vi "RF Characterization UI Merged.vi"() -> ()   [LabVIEW 2010]
uses:
  RF Characterization States.ctl
  Drivers/Motion/Motion_Gantry Position.ctl
  <vilib>/Utility/NIReport.llb/NI_report.lvclass
  Report Generation States.ctl
  <vilib>/Analysis/1siggen.llb/Ramp Pattern by Delta.vi
  <vilib>/Utility/NIReport.llb/Append Text Table to Report (wrap).vi
  <vilib>/Utility/NIReport.llb/Append Numeric Table to Report (wrap).vi
  <vilib>/Analysis/NI_AALBase.lvlib
panel:
  in  "Close":bool
  in  "stop":bool
  in  "Prev":bool
  in  "Next":bool
  out "Main Tab Control":T1(tab)
  out "Gantry Moving Message":string="Gantry Moving"
  in  "Z":dbl min=-5.5 max=5.5 step=0.001 format="%.3g"
  in  "Y":dbl min=-5.5 max=5.5 step=0.001 format="%.3g"
  in  "X":dbl min=0.0 max=22.0 step=0.001 format="%.3g"
  in  "Gantry TCP address:port":string="192.168.0.3:502"
  in  "MICS ID":u32 format="%06.0x"
  in  "MICS Dongle Port":refnum<visa-resource-name>="COM5"
  in  "Start Attenuation Test":bool
  in  "Attenuation Samples":i32(knob)=1 caption="Samples" min=1 max=30 step=1 scale=1.0..30.0
  in  "Attenuation Increment":dbl(knob)=0.25 caption="Increment" min=0.25 max=5.0 step=0.25 scale=0.25..5.0
  in  "Attenuation Range":cluster{dbl, dbl}(slide)={0.0, 1.4141414141414141} caption="Range" scale=0.0..30.0
  out "Attenuation Graph":cluster{dbl, dbl}[](graph)
  out "Attenuation Cutoff (dB)":dbl=12.5
  out "MICS Power Graph":cluster{dbl, dbl}[](graph)
  in  "Power Range":cluster{dbl, dbl}(slide) caption="Range" scale=0.0..64.0
  in  "Power Increment":dbl(knob)=1.0 caption="Increment" min=1.0 max=5.0 step=1.0 scale=1.0..5.0
  in  "Power Samples":i32(knob)=1 caption="Samples" min=1 max=30 step=1 scale=1.0..30.0
  in  "Start Power Test":bool
  out "Power Cutoff":i32=12 format="%.0x"
  in  "Z-Layer":dbl(slide) min=0.0 max=0.0 step=1.0 scale=-5.5..5.5
  in  "X Range":cluster{"Min":dbl, "Max":dbl, "Increment":dbl}={"Min"=1.0, "Max"=20.0, "Increment"=0.25}
  in  "Y Range":cluster{"Min":dbl, "Max":dbl, "Increment":dbl}={"Min"=-5.0, "Max"=5.0, "Increment"=0.25}
  in  "Z Range":cluster{"Min":dbl, "Max":dbl, "Increment":dbl}={"Min"=0.0, "Max"=0.0, "Increment"=1.0}
  out "RF Mapping Graph":dbl[][](graph)
  in  "Mapping Samples":i32(knob)=1 caption="Samples" min=1 max=30 step=1 scale=1.0..30.0
  in  "Start RF Mapping":bool
  in  "WebBrowser":refnum<k7>(container)
  in  "Save Report":bool
  # "Gantry Configuration"
  # "MICS Configuration"
  # "Instructions:"
  # "Instructions:"
  # "Instructions:\nLorem ipsum veritas quo\nLorem ipsum veritas quo\nLorem ipsum veritas quo\nLorem ipsum veritas quo\nLorem ipsum veritas quo\nLorem ipsum veritas quo\nLorem ipsum veritas quo\nLorem ipsum veritas quo\nLorem ipsum veritas quo"
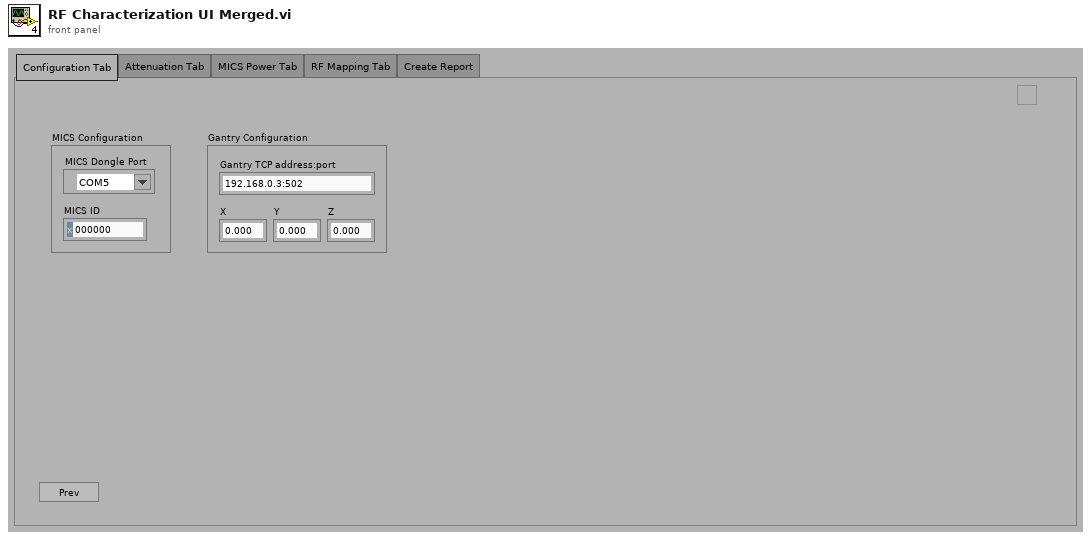
[diagram p1: front panel]
types:
  T1 = enum32{"Configuration Tab", "Attenuation Tab", "MICS Power Tab", "RF Mapping Tab", "Create Report"}
  T2 = typedef "RF Characterization States.ctl" = enum16{"Initialize", "Enable/Disable Navigation", "Set Next Action", "Set Prev Action", "Set Stop Action", "Prev Action Triggered", "Next Action Triggered", "Stop Action Triggered", "Move Gantry to Position", "Display Configuration Tab", "Check Configuration", "Display Attenuation Tab", "Check Attenuation Config", "Start Attenuation Test", "Check Attenuation Results", "Display Power Tab", "Check Power Config", "Start Power Test", "Check Power Results", "Display Mapping Tab", "Check Mapping Config", "Start Mapping Test", "Take Mapping Sample", "Finish Mapping Test", "Check Mapping Results", "Display Report Tab", "Generate Report", "Save Report", "Error", "Shutdown"}
  T3 = typedef "Motion_Gantry Position.ctl" = cluster{"Gantry Accel/Decel":dbl, "Gantry Velocity":dbl, "X-Position":dbl, "Y-Position":dbl, "Z-Position":dbl}
  T4 = cluster{"Next Action":cluster{"Action":T2, "Payload":variant}, "Prev Action":cluster{"Action":T2, "Payload":variant}, "Stop Action":cluster{"Action":T2, "Payload":variant}, "Configuration":cluster{"MICS Dongle Port":refnum<visa-resource-name>, "MICS ID":u32, "Gantry TCP address:port":string, "X-Position":dbl, "Y-Position":dbl, "Z-Position":dbl}, "Attenuation Config":cluster{"Range":cluster{dbl, dbl}, "Increment":dbl, "Samples":i32}, "Attenuation Results":cluster{dbl, dbl}[], "Attenuation Cutoff (dB)":dbl, "Power Config":cluster{"Range":cluster{dbl, dbl}, "Increment":dbl, "Samples":i32}, "Power Results":cluster{dbl, dbl}[], "Power Cutoff":u8, "Mapping Config":cluster{"Samples":i32, "X Range":cluster{"Min":dbl, "Max":dbl, "Increment":dbl}, "Y Range":cluster{"Min":dbl, "Max":dbl, "Increment":dbl}, "Z Range":cluster{"Min":dbl, "Max":dbl, "Increment":dbl}, "Positions":T3[], "Indices":cluster{i32, i32, i32}[]}, "Mapping Results":dbl[][][], "Refnums":cluster{"MICS Refnum":refnum<visa-resource-name>, "Motion Refnum":refnum<k5>}, "Mapping Index":i32, "Temp Report Path":path, "Previous Start Path":path, "Report":refnum<class "NI_report.lvclass">}
  T5 = enum8{"Enabled", "Disabled", "Disabled and Grayed Out"}
  T6 = cluster{"Prev Button":cluster{"Visible":bool, "Enable":enum8{"Enabled", "Disabled", "Disabled and Grayed Out"}}, "Next Button":cluster{"Visible":bool, "Enable":enum8{"Enabled", "Disabled", "Disabled and Grayed Out"}}, "Stop Button":cluster{"Visible":bool, "Enable":enum8{"Enabled", "Disabled", "Disabled and Grayed Out"}}}
  T7 = enum32{"Configuration Tab", "Attenuation Tab", "MICS Power Tab", "RF Mapping Tab"}
  T8 = typedef "Report Generation States.ctl" = enum16{"Initialize", "Generate Header", "Generate Summary", "Generate Attenuation Section", "Generate MICS Power Section", "Generate RF Mapping Section 1", "Generate RF Mapping Section 2", "Show Report in UI"}
  T9 = enum16{"Standard Report", "HTML", "Word", "Excel"}
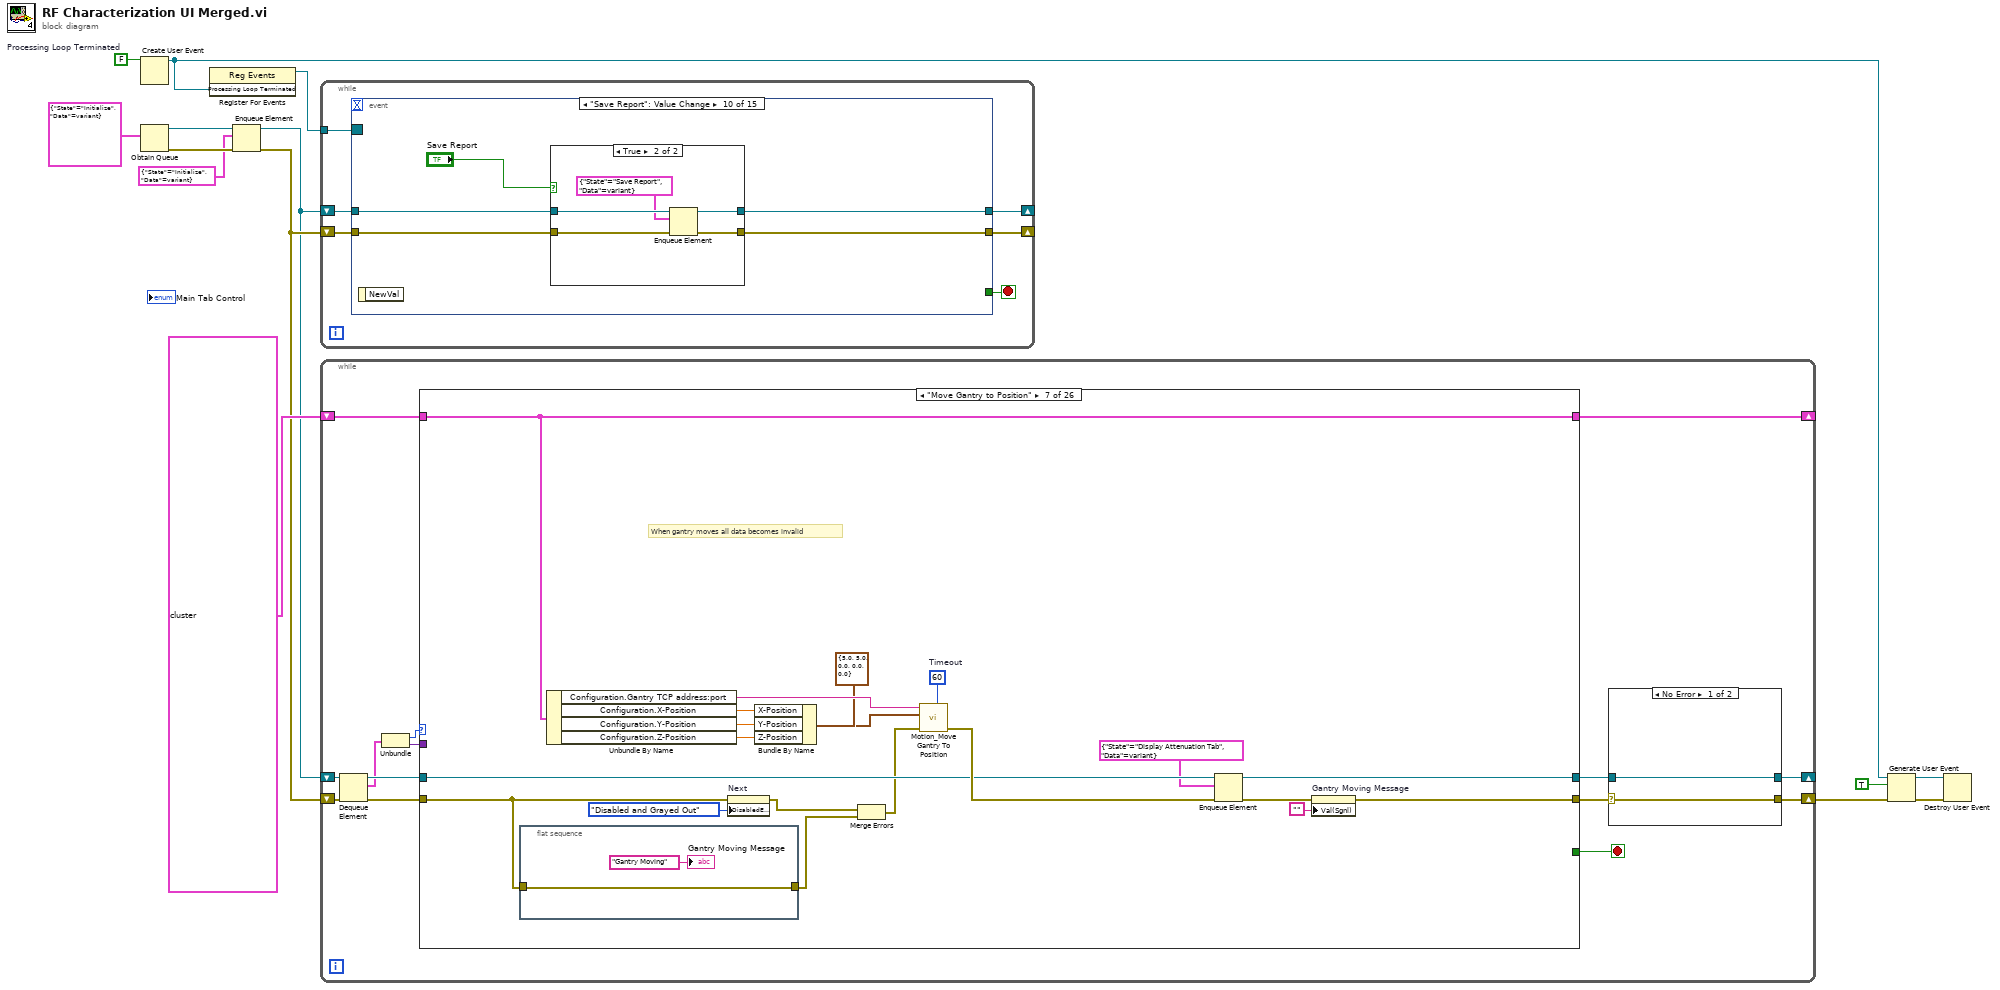
[diagram p0: block diagram]
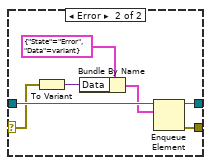
[diagram p2: hidden frame]
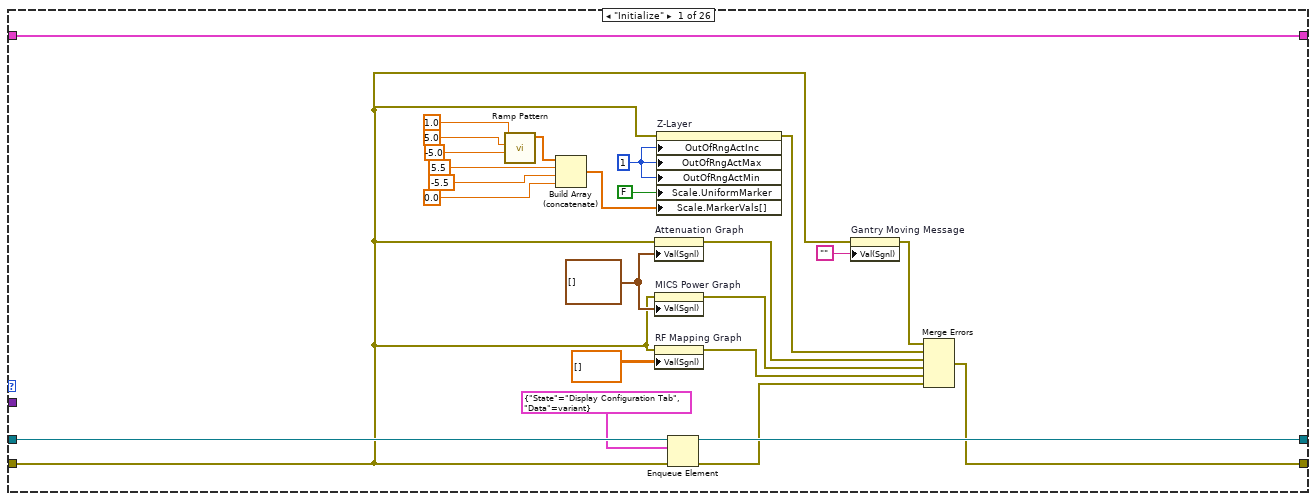
[diagram p3: hidden frame]
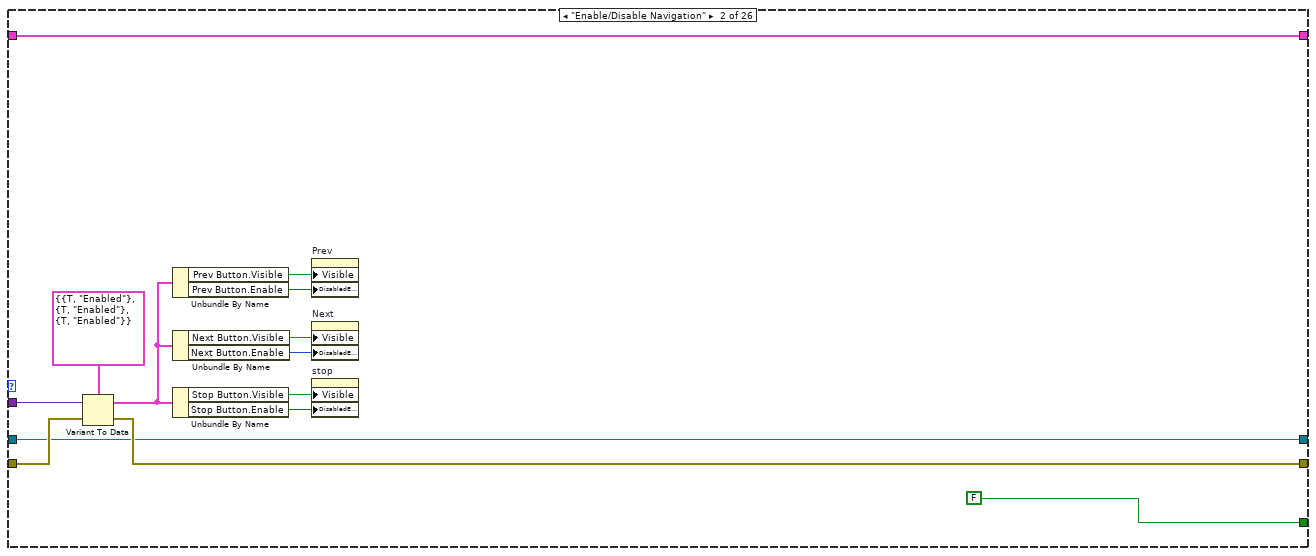
[diagram p4: hidden frame]
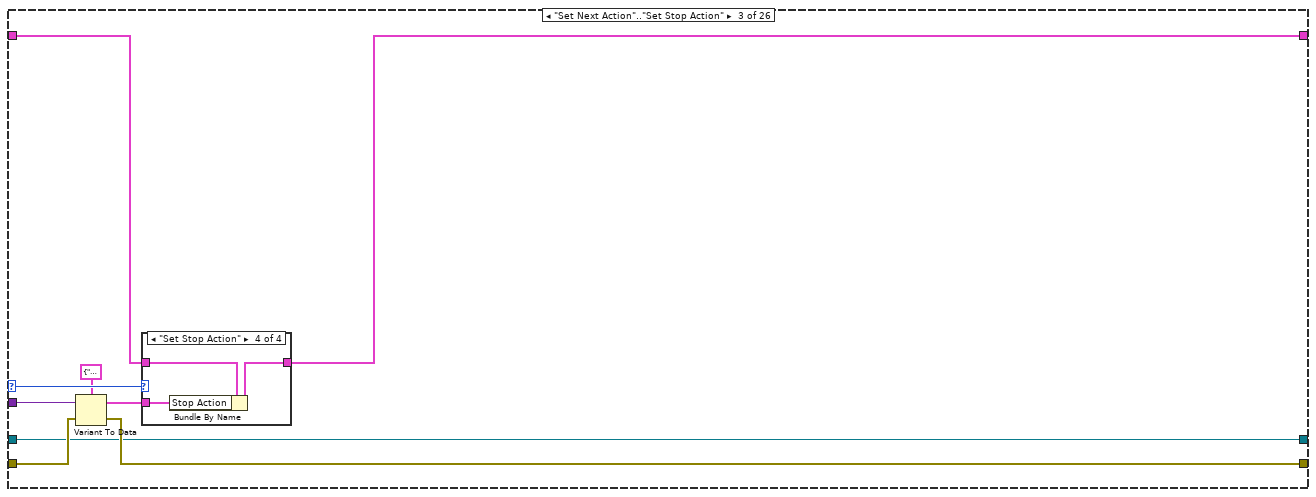
[diagram p5: hidden frame]
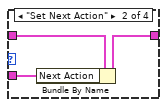
[diagram p7: hidden frame]
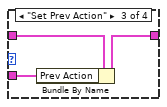
[diagram p8: hidden frame]
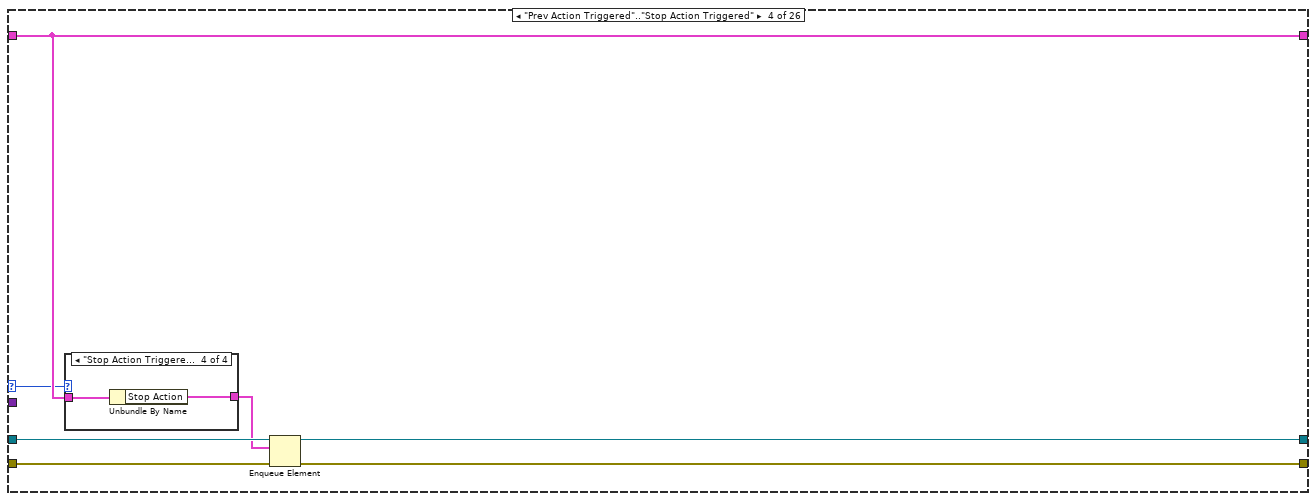
[diagram p9: hidden frame]
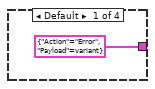
[diagram p10: hidden frame]
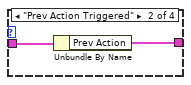
[diagram p11: hidden frame]
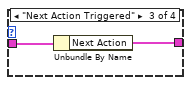
[diagram p12: hidden frame]
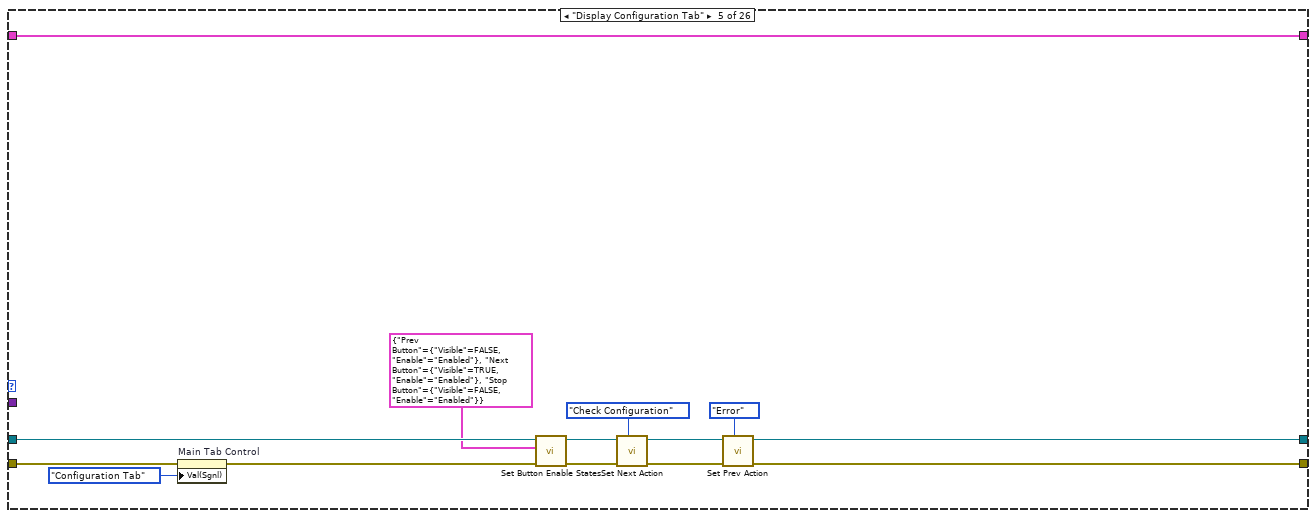
[diagram p13: hidden frame]
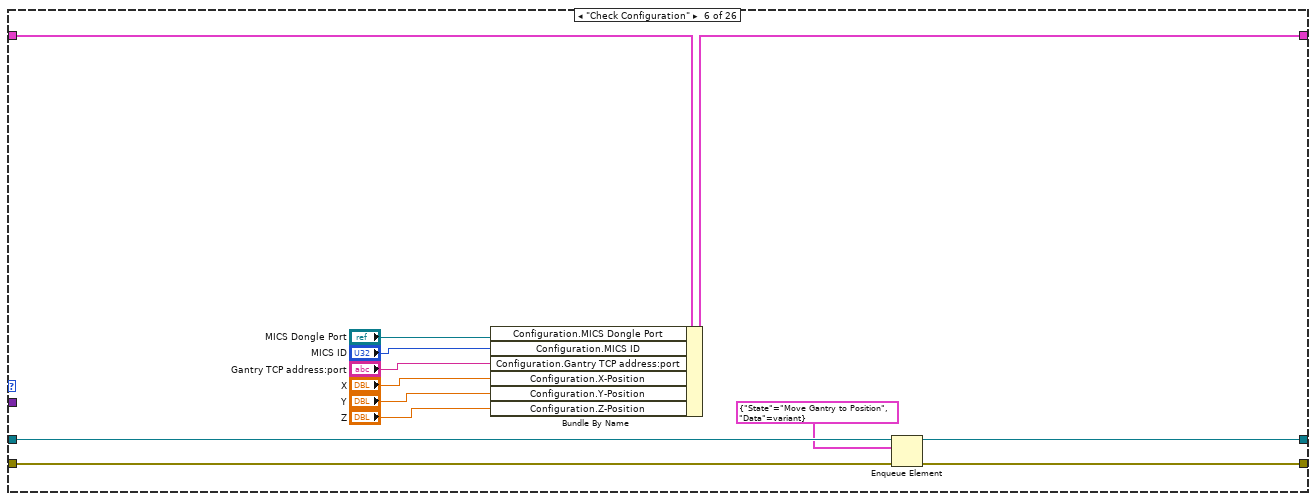
[diagram p14: hidden frame]
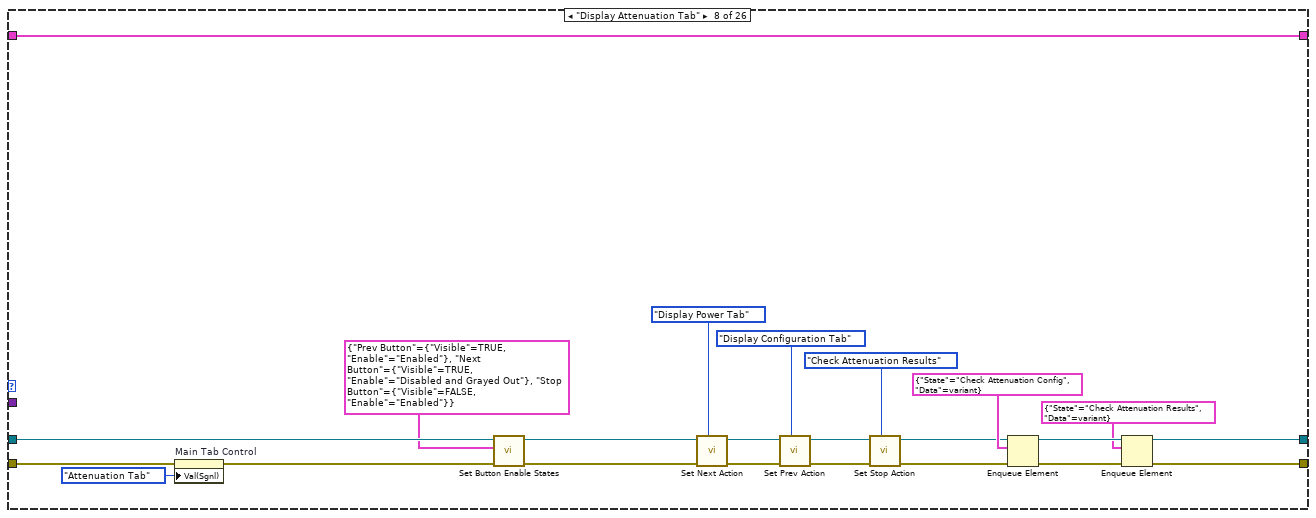
[diagram p15: hidden frame]
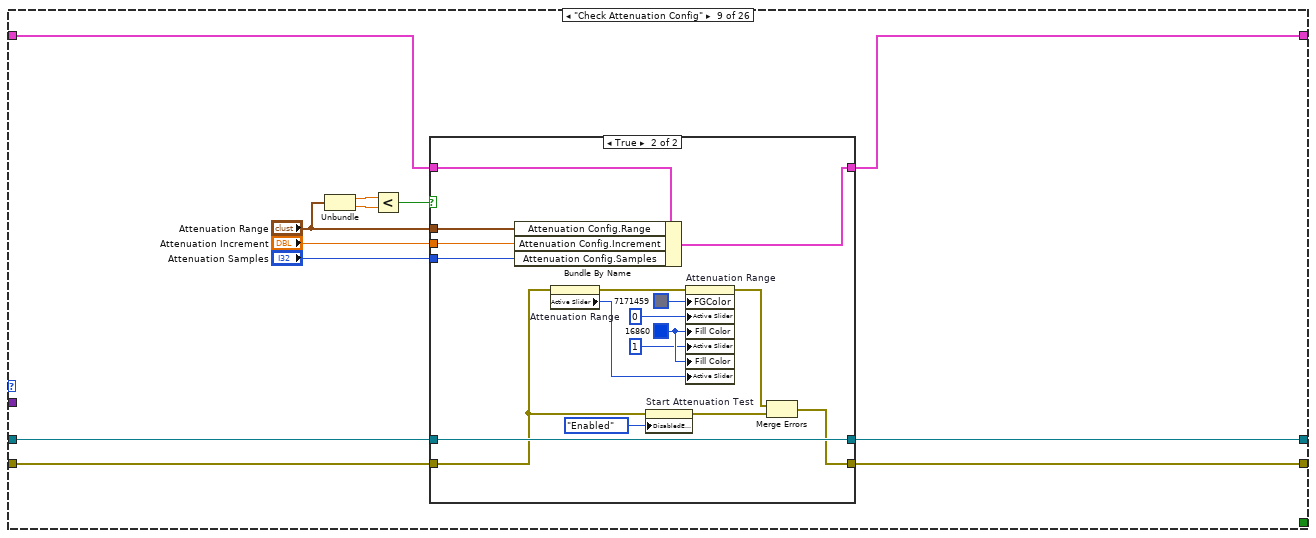
[diagram p16: hidden frame]
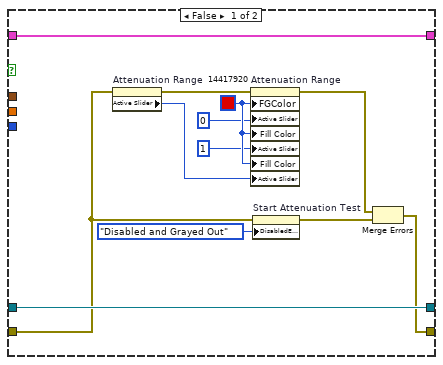
[diagram p17: hidden frame]
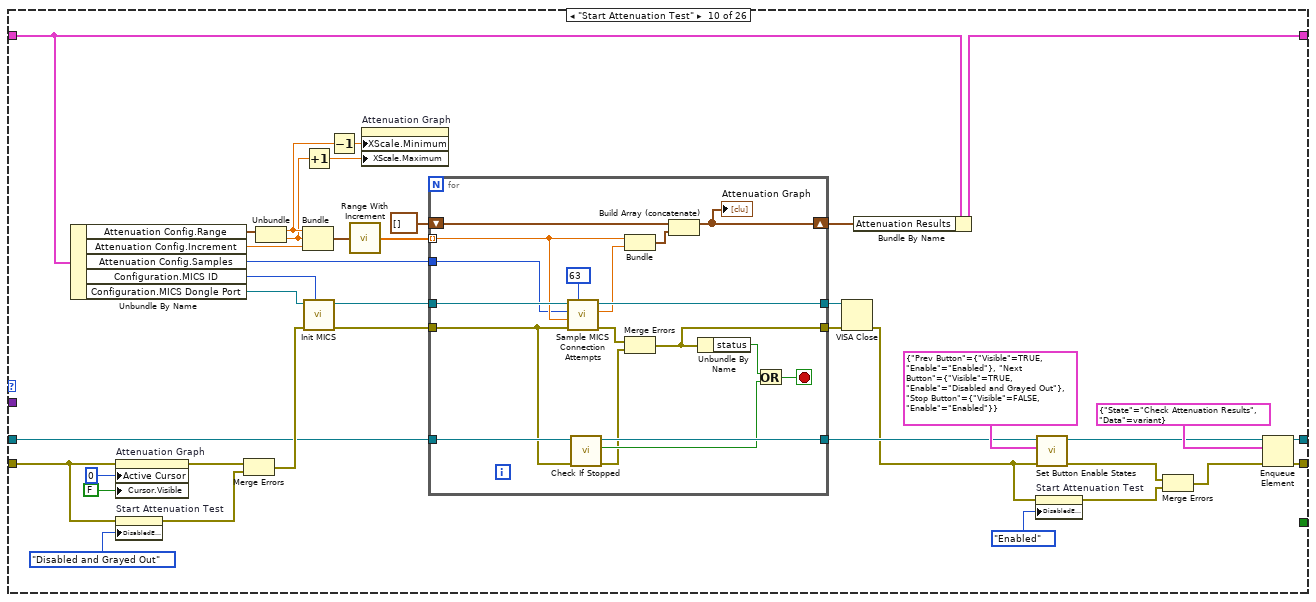
[diagram p18: hidden frame]
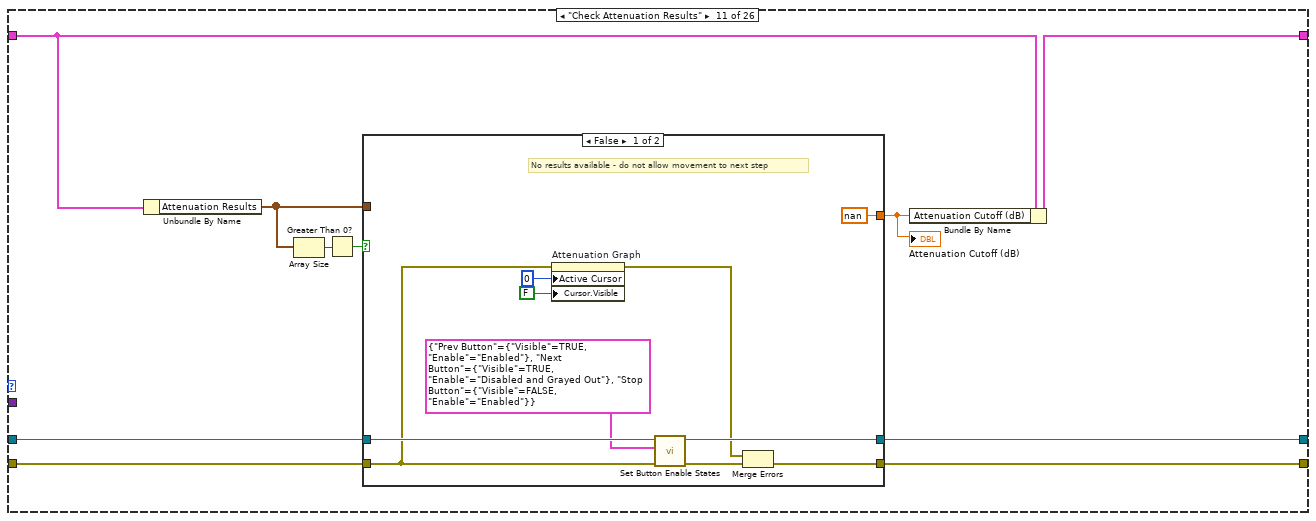
[diagram p19: hidden frame]
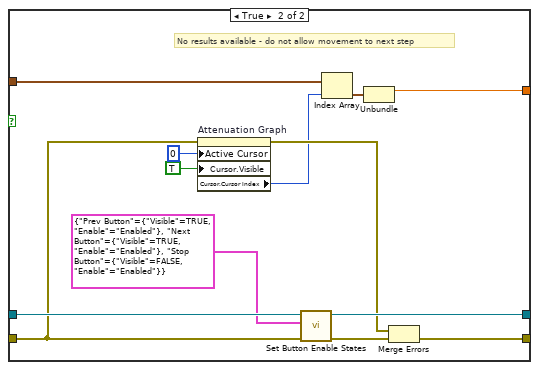
[diagram p20: hidden frame]
diagram:
  w11 = FALSE  # Processing Loop Terminated
  n1 = Create User Event(user event datatype=w11) -> (user event=w8:refnum<user-event>)  [unwired: 1 in, 1 out]
  n2 = Obtain Queue(element data type=cluster{"State":T2, "Data":variant} {"State"=enum."Initialize", "Data"=variant}) -> (queue out=w3:refnum<queue>, error out=w12:errorcluster)  [unwired: 4 in, 1 out]
  n3 = register-events(w8) -> (reference out=w10:refnum<event-registration>)  [unwired: 2 in, 1 out]
  n4 = Enqueue Element(queue=w3, element=cluster{"State":T2, "Data":variant} {"State"=enum."Initialize", "Data"=variant}, error in (no error)=w12) -> (queue out=w2:refnum<queue>, error out=w4:errorcluster)  [unwired: 1 in, 1 out]
  n5 = while {
    shift-right: [w19] -> _
    shift-left: w2 -> [w20]
    shift-right: [w17] -> _
    shift-left: w4 -> [w18]
    tunnel: w10 -> [w16]
    stop <- w15 stop-if-true
    n6 = event shown="[9] \"Save Report\": Value Change" {
      selector: w16 -> [_ _ _ _ _ _ _ _ _ _ _ _ _ _ _]
      dyn-events: _ -> [_ _ _ _ _ _ _ _ _ _ _ _ _ _ _]
      timeout: _ -> [_ _ _ _ _ _ _ _ _ _ _ _ _ _ _]
      tunnel: w20 -> [w22 w24 w30 w43 w55 w67 w80 w96 w107 w120 w132 w137 w141 w145 w150]
      tunnel: [w22 w24 w28 w41 w54 w65 w77 w93 w105 w118 w129 w134 w139 w144 w149] -> w19
      tunnel: w18 -> [w21 w23 w29 w40 w53 w66 w78 w94 w106 w119 w130 w135 w140 w147 w152]
      tunnel: [w21 w23 w27 w39 w52 w64 w79 w95 w104 w117 w131 w136 w138 w146 w151] -> w17
      tunnel: [_ w25 TRUE ("Processing Loop Terminated") _ _ _ _ _ _ _ _ _ _ _ _] -> w15
      event Timeout {
        n7 = event-data() -> ()  [unwired: 1 in, 2 out]
      }
      event User Event {
        n8 = event-data() -> ("Processing Loop Terminated"=w25:bool)  [unwired: 1 in, 3 out]
      }
      event "Close": Value Change {
        n9 = event-data() -> ()  [unwired: 1 in, 1 out]
        n10 = case shown="True" "Close" {
          tunnel: w30 -> [w33 w37]
          tunnel: w29 -> [w32 w38]
          tunnel: [w33 w36] -> w28
          tunnel: [w32 w35] -> w27
          frame False {
          }
          frame True {
            n11 = Enqueue Element(queue=w37, element=cluster{"State":T2, "Data":variant} {"State"=enum."Shutdown", "Data"=variant}, error in (no error)=w38) -> (queue out=w36:refnum<queue>, error out=w35:errorcluster)  [unwired: 1 in, 1 out]
          }
        }
      }
      event "Next": Value Change {
        n12 = event-data() -> ()  [unwired: 1 in, 1 out]
        n13 = case shown="True" "Next" {
          tunnel: w43 -> [w45 w50]
          tunnel: [w45 w49] -> w41
          tunnel: w40 -> [w44 w48]
          tunnel: [w44 w47] -> w39
          frame False {
          }
          frame True {
            n14 = Enqueue Element(queue=w50, element=cluster{"State":T2, "Data":variant} {"State"=enum."Next Action Triggered", "Data"=variant}, error in (no error)=w48) -> (queue out=w49:refnum<queue>, error out=w47:errorcluster)  [unwired: 1 in, 1 out]
          }
        }
      }
      event "Prev": Value Change {
        n15 = event-data() -> ()  [unwired: 1 in, 1 out]
        n16 = case shown="True" "Prev" {
          tunnel: w55 -> [w57 w62]
          tunnel: [w57 w61] -> w54
          tunnel: w53 -> [w56 w60]
          tunnel: [w56 w59] -> w52
          frame False {
          }
          frame True {
            n17 = Enqueue Element(queue=w62, element=cluster{"State":T2, "Data":variant} {"State"=enum."Prev Action Triggered", "Data"=variant}, error in (no error)=w60) -> (queue out=w61:refnum<queue>, error out=w59:errorcluster)  [unwired: 1 in, 1 out]
          }
        }
      }
      event "stop": Value Change {
        n18 = event-data() -> ()  [unwired: 1 in, 1 out]
        n19 = case shown="True" "stop" {
          tunnel: w67 -> [w69 w76]
          tunnel: [w69 w75] -> w65
          tunnel: w66 -> [w68 w74]
          tunnel: [w68 w71] -> w64
          frame False {
          }
          frame True {
            n20 = Enqueue Element(queue=w76, element=cluster{"State":T2, "Data":variant} {"State"=enum."Stop Action Triggered", "Data"=variant}, error in (no error)=w74) -> (queue out=w75:refnum<queue>, error out=w72:errorcluster)  [unwired: 1 in, 1 out]
            n21 = property on="stop" class="Bool"(error in=w72, "DisabledEnum"=T5."Disabled and Grayed Out" ("Disabled")) -> (error out=w71:errorcluster)  [unwired: 1 in, 1 out]
          }
        }
      }
      event "Start Attenuation Test": Value Change {
        n22 = event-data() -> ()  [unwired: 1 in, 1 out]
        n23 = case shown="True" "Start Attenuation Test" {
          tunnel: w80 -> [w83 w88]
          tunnel: [w82 w91] -> w79
          tunnel: w78 -> [w82 w87]
          tunnel: [w83 w90] -> w77
          frame False {
          }
          frame True {
            n24 = call "Set Button Enable States.vi"("error in (no error)"=w87, "Button States"=T6 {"Prev Button"={"Visible"=TRUE, "Enable"=enum."Disabled and Grayed Out"}, "Next Button"={"Visible"=TRUE, "Enable"=enum."Disabled and Grayed Out"}, "Stop Button"={"Visible"=TRUE, "Enable"=enum."Enabled"}}, "queue in"=w88) -> ("error out"=w85:errorcluster, "queue out"=w86:refnum<queue>)  [unwired: 7 in]
            n25 = Enqueue Element(queue=w86, element=cluster{"State":T2, "Data":variant} {"State"=enum."Start Attenuation Test", "Data"=variant}, error in (no error)=w85) -> (queue out=w90:refnum<queue>, error out=w91:errorcluster)  [unwired: 1 in, 1 out]
          }
        }
      }
      event "Start Power Test": Value Change {
        n26 = event-data() -> ()  [unwired: 1 in, 1 out]
        n27 = case shown="True" "Start Power Test" {
          tunnel: w96 -> [w98 w101]
          tunnel: [w97 w102] -> w95
          tunnel: w94 -> [w97 w103]
          tunnel: [w98 w100] -> w93
          frame False {
          }
          frame True {
            n28 = Enqueue Element(queue=w101, element=cluster{"State":T2, "Data":variant} {"State"=enum."Start Power Test", "Data"=variant}, error in (no error)=w103) -> (queue out=w100:refnum<queue>, error out=w102:errorcluster)  [unwired: 1 in, 1 out]
          }
        }
      }
      event "Start RF Mapping": Value Change {
        n29 = event-data() -> ()  [unwired: 1 in, 1 out]
        n30 = case shown="True" "Start RF Mapping" {
          tunnel: w107 -> [w110 w115]
          tunnel: w106 -> [w109 w114]
          tunnel: [w110 w112] -> w105
          tunnel: [w109 w111] -> w104
          frame False {
          }
          frame True {
            n31 = Enqueue Element(queue=w115, element=cluster{"State":T2, "Data":variant} {"State"=enum."Start Mapping Test", "Data"=variant}, error in (no error)=w114) -> (queue out=w112:refnum<queue>, error out=w111:errorcluster)  [unwired: 1 in, 1 out]
          }
        }
      }
      event "Save Report": Value Change {
        n32 = event-data() -> ()  [unwired: 1 in, 1 out]
        n33 = case shown="True" "Save Report" {
          tunnel: w120 -> [w122 w127]
          tunnel: w119 -> [w121 w126]
          tunnel: [w122 w124] -> w118
          tunnel: [w121 w123] -> w117
          frame False {
          }
          frame True {
            n34 = Enqueue Element(queue=w127, element=cluster{"State":T2, "Data":variant} {"State"=enum."Save Report", "Data"=variant}, error in (no error)=w126) -> (queue out=w124:refnum<queue>, error out=w123:errorcluster)  [unwired: 1 in, 1 out]
          }
        }
      }
      event "Attenuation Range", "Attenuation Increment", "Attenuation Samples": Value Change {
        n35 = event-data() -> ()  [unwired: 1 in, 1 out]
        n36 = Enqueue Element(queue=w132, element=cluster{"State":T2, "Data":variant} {"State"=enum."Check Attenuation Config", "Data"=variant}, error in (no error)=w130) -> (queue out=w129:refnum<queue>, error out=w131:errorcluster)  [unwired: 1 in, 1 out]
      }
      event "Attenuation Graph": Cursor Move {
        n37 = event-data() -> ()  [unwired: 1 in, 1 out]
        n38 = Enqueue Element(queue=w137, element=cluster{"State":T2, "Data":variant} {"State"=enum."Check Attenuation Results", "Data"=variant}, error in (no error)=w135) -> (queue out=w134:refnum<queue>, error out=w136:errorcluster)  [unwired: 1 in, 1 out]
      }
      event "Power Range", "Power Increment", "Power Samples": Value Change {
        n39 = event-data() -> ()  [unwired: 1 in, 1 out]
        n40 = Enqueue Element(queue=w141, element=cluster{"State":T2, "Data":variant} {"State"=enum."Check Power Config", "Data"=variant}, error in (no error)=w140) -> (queue out=w139:refnum<queue>, error out=w138:errorcluster)  [unwired: 1 in, 1 out]
      }
      event "MICS Power Graph": Cursor Move {
        n41 = event-data() -> ()  [unwired: 1 in, 1 out]
        n42 = Enqueue Element(queue=w145, element=cluster{"State":T2, "Data":variant} {"State"=enum."Check Power Results", "Data"=variant}, error in (no error)=w147) -> (queue out=w144:refnum<queue>, error out=w146:errorcluster)  [unwired: 1 in, 1 out]
      }
      event "Z-Layer": Value Change {
        n43 = event-data() -> ()  [unwired: 1 in, 1 out]
        n44 = Enqueue Element(queue=w150, element=cluster{"State":T2, "Data":variant} {"State"=enum."Check Mapping Results", "Data"=variant}, error in (no error)=w152) -> (queue out=w149:refnum<queue>, error out=w151:errorcluster)  [unwired: 1 in, 1 out]
      }
    }
  }
  n45 = while {
    shift-right: [w154] -> w9
    shift-left: w4 -> [w165]
    shift-right: [w153] -> _
    shift-left: w2 -> [w166]
    shift-right: [w159] -> _
    shift-left: T4 {"Next Action"={"Action"=enum."Error", "Payload"=variant}, "Prev Action"={"Action"=enum."Error", "Payload"=variant}, "Stop Action"={"Action"=enum."Error", "Payload"=variant}, "Configuration"={"MICS Dongle Port"="", "MICS ID"=0, "Gantry TCP address:port"="", "X-Position"=0.0, "Y-Position"=0.0, "Z-Position"=0.0}, "Attenuation Config"={"Range"={0.0, 0.0}, "Increment"=0.0, "Samples"=0}, "Attenuation Results"=[], "Attenuation Cutoff (dB)"=0.0, "Power Config"={"Range"={0.0, 0.0}, "Increment"=0.0, "Samples"=0}, "Power Results"=[], "Power Cutoff"=0, "Mapping Config"={"Samples"=0, "X Range"={"Min"=0.0, "Max"=0.0, "Increment"=0.0}, "Y Range"={"Min"=0.0, "Max"=0.0, "Increment"=0.0}, "Z Range"={"Min"=0.0, "Max"=0.0, "Increment"=0.0}, "Positions"=[], "Indices"=[]}, "Mapping Results"=[], "Refnums"={"MICS Refnum"="", "Motion Refnum"=refnum}, "Mapping Index"=0, "Temp Report Path"=path "", "Previous Start Path"=path "", "Report"=refnum} -> [w160]
    stop <- w157 stop-if-true
    n46 = Dequeue Element(queue=w166, error in (no error)=w165) -> (queue out=w164:refnum<queue>, element=w163:cluster{"State":T2, "Data":variant}, error out=w158:errorcluster)  [unwired: 1 in, 1 out]
    n47 = Unbundle(w163) -> ("State"=w162:T2, "Data"=w161:variant)
    n48 = case shown="\"Move Gantry to Position\"" w162 {
      selector: w162 -> [_ _ w218 w234 _ _ _ _ _ _ _ _ _ _ _ _ _ _ _ _ _ _ _ _ _ _]
      tunnel: [w191 w207 w221 w235 w255 w265 w276 w305 w320 w383 w421 w450 w478 w538 w576 w606 w629 w643 w694 w726 w751 w756 w777 w1010 w1044 w1054] -> w156
      tunnel: w164 -> [w199 w206 w217 w240 w252 w264 w291 w315 w323 w362 w424 w452 w481 w517 w579 w609 w630 w642 w687 w732 w752 w760 w779 w1009 w1043 w1055]
      tunnel: w161 -> [_ w213 w223 _ _ _ _ _ _ _ _ _ _ _ _ _ _ _ _ _ _ _ _ _ w1041 _]
      tunnel: [_ FALSE _ _ _ _ _ _ _ _ _ _ _ _ _ _ _ _ _ _ _ _ _ _ _ TRUE] -> w157
      tunnel: [w198 w206 w217 w236 w257 w263 w290 w303 w321 w382 w422 w451 w479 w537 w577 w607 w630 w644 w693 w727 w752 w754 w779 w1009 w1042 w1055] -> w155
      tunnel: w160 -> [w200 w205 w220 w238 w261 w268 w294 w319 w329 w385 w419 w472 w474 w540 w574 w628 w631 w654 w709 w737 w749 w757 w774 w1020 w1045 w1056]
      tunnel: [w200 w205 w219 w238 w261 w267 w294 w319 w328 w384 w418 w472 w473 w539 w573 w628 w631 w636 w708 w737 w749 w757 w778 w1020 w1045 w1056] -> w159
      tunnel: w158 -> [w178 w208 w222 w239 w259 w266 w281 w318 w322 w361 w423 w453 w480 w516 w578 w608 w629 w650 w715 w735 w751 w770 w776 w1018 w1039 w1054]
      frame "Initialize" {
        w190 = u8 1 ("Response to Value Outside Limits:Increment")
        w196 = cluster{dbl, dbl}[] [] ("Value (Signaling)")
        n49 = call-poly <vilib>:"Ramp Pattern.vi"("start"=-5.0, "end"=5.0, "delta"=1.0) -> ("Ramp Pattern"=w188:dbl[])  [unwired: 6 in, 2 out]
        n50 = Build Array (concatenate)(w188, 5.5 ("delta"), -5.5 ("delta"), 0.0 ("delta")) -> (w181:dbl[])
        n51 = property on="Attenuation Graph" class="XYGraph (strict)"(error in=w178, "Val(Sgnl)"=w196) -> (error out=w177:errorcluster)  [unwired: 1 in, 1 out]
        n52 = property on="MICS Power Graph" class="XYGraph (strict)"(error in=w178, "Val(Sgnl)"=w196) -> (error out=w193:errorcluster)  [unwired: 1 in, 1 out]
        n53 = property on="RF Mapping Graph" class="IntGraph (strict)"(error in=w178, "Val(Sgnl)"=dbl[][] [] ("Value (Signaling)")) -> (error out=w194:errorcluster)  [unwired: 1 in, 1 out]
        n54 = property on="Z-Layer" class="Slide (strict)"(error in=w178, "OutOfRngActInc"=w190, "OutOfRngActMax"=w190, "OutOfRngActMin"=w190, "Scale.UniformMarker"=FALSE ("Scale.Uniform Marker Spacing?"), "Scale.MarkerVals[]"=w181) -> (error out=w180:errorcluster)  [unwired: 1 in, 1 out]
        n55 = Enqueue Element(queue=w199, element=cluster{"State":T2, "Data":variant} {"State"=enum."Display Configuration Tab", "Data"=variant}, error in (no error)=w178) -> (queue out=w198:refnum<queue>, error out=w192:errorcluster)  [unwired: 1 in, 1 out]
        n56 = property on="Gantry Moving Message" class="Str"(error in=w178, "Val(Sgnl)"="") -> (error out=w179:errorcluster)  [unwired: 1 in, 1 out]
        n57 = Merge Errors(w179, w180, w177, w193, w194, w192) -> (w191:errorcluster)
      }
      frame "Enable/Disable Navigation" {
        n58 = Variant To Data(error in=w208, Variant=w213, type=T6 {"Prev Button"={"Visible"=TRUE, "Enable"=enum."Enabled"}, "Next Button"={"Visible"=TRUE, "Enable"=enum."Enabled"}, "Stop Button"={"Visible"=TRUE, "Enable"=enum."Enabled"}} ("Button States")) -> (error out=w207:errorcluster, data=w203:T6)
        n59 = Unbundle By Name(w203) -> ("Prev Button.Visible"=w212:bool, "Prev Button.Enable"=w211:T5)
        n60 = Unbundle By Name(w203) -> ("Next Button.Visible"=w210:bool, "Next Button.Enable"=w209:T5)
        n61 = Unbundle By Name(w203) -> ("Stop Button.Visible"=w202:bool, "Stop Button.Enable"=w201:T5)
        n62 = property on="Prev" class="Bool"("Visible"=w212, "DisabledEnum"=w211) -> ()  [unwired: 2 in, 2 out]
        n63 = property on="Next" class="Bool"("Visible"=w210, "DisabledEnum"=w209) -> ()  [unwired: 2 in, 2 out]
        n64 = property on="stop" class="Bool"("Visible"=w202, "DisabledEnum"=w201) -> ()  [unwired: 2 in, 2 out]
      }
      frame "Set Next Action".."Set Stop Action" {
        n65 = Variant To Data(error in=w222, Variant=w223, type=cluster{"Action":T2, "Payload":variant} {"Action"=enum."Error", "Payload"=variant} ("Action")) -> (error out=w221:errorcluster, data=w215:cluster{"Action":T2, "Payload":variant})
        n66 = case shown="\"Set Stop Action\"" w218 {
          tunnel: w215 -> [_ w227 w230 w233]
          tunnel: w220 -> [w224 w226 w229 w232]
          tunnel: [w224 w225 w228 w231] -> w219
          frame Default {
          }
          frame "Set Next Action" {
            n67 = Bundle By Name(cluster=w226, "Next Action"=w227) -> (w225:T4)
          }
          frame "Set Prev Action" {
            n68 = Bundle By Name(cluster=w229, "Prev Action"=w230) -> (w228:T4)
          }
          frame "Set Stop Action" {
            n69 = Bundle By Name(cluster=w232, "Stop Action"=w233) -> (w231:T4)
          }
        }
      }
      frame "Prev Action Triggered".."Stop Action Triggered" {
        n70 = case shown="\"Stop Action Triggered\"" w234 {
          tunnel: w238 -> [_ w243 w245 w247]
          tunnel: [cluster{"Action":T2, "Payload":variant} {"Action"=enum."Error", "Payload"=variant} ("Prev Action") w242 w244 w246] -> w237
          frame Default {
          }
          frame "Prev Action Triggered" {
            n71 = Unbundle By Name(w243) -> ("Prev Action"=w242:cluster{"Action":T2, "Payload":variant})
          }
          frame "Next Action Triggered" {
            n72 = Unbundle By Name(w245) -> ("Next Action"=w244:cluster{"Action":T2, "Payload":variant})
          }
          frame "Stop Action Triggered" {
            n73 = Unbundle By Name(w247) -> ("Stop Action"=w246:cluster{"Action":T2, "Payload":variant})
          }
        }
        n74 = Enqueue Element(queue=w240, element=w237, error in (no error)=w239) -> (queue out=w236:refnum<queue>, error out=w235:errorcluster)  [unwired: 1 in, 1 out]
      }
      frame "Display Configuration Tab" {
        n75 = property on="Main Tab Control" class="TabCtl (strict)"(error in=w259, "Val(Sgnl)"=T7."Configuration Tab" ("Value (Signaling)")) -> (error out=w251:errorcluster)  [unwired: 1 in, 1 out]
        n76 = call "Set Button Enable States.vi"("error in (no error)"=w251, "Button States"=T6 {"Prev Button"={"Visible"=FALSE, "Enable"=enum."Enabled"}, "Next Button"={"Visible"=TRUE, "Enable"=enum."Enabled"}, "Stop Button"={"Visible"=FALSE, "Enable"=enum."Enabled"}}, "queue in"=w252) -> ("error out"=w250:errorcluster, "queue out"=w249:refnum<queue>)  [unwired: 7 in]
        n77 = call "Set Next Action.vi"("Action"=RF_Characterization_States."Check Configuration", "error in (no error)"=w250, "queue in"=w249) -> ("error out"=w256:errorcluster, "queue out"=w258:refnum<queue>)  [unwired: 7 in]
        n78 = call "Set Prev Action.vi"("Action"=RF_Characterization_States."Error", "error in (no error)"=w256, "queue in"=w258) -> ("error out"=w255:errorcluster, "queue out"=w257:refnum<queue>)  [unwired: 7 in]
      }
      frame "Check Configuration" {
        n79 = Bundle By Name(cluster=w268, "Configuration.MICS Dongle Port"="MICS Dongle Port", "Configuration.MICS ID"="MICS ID", "Configuration.Gantry TCP address:port"="Gantry TCP address:port", "Configuration.X-Position"="X", "Configuration.Y-Position"="Y", "Configuration.Z-Position"="Z") -> (w267:T4)
        n80 = Enqueue Element(queue=w264, element=cluster{"State":T2, "Data":variant} {"State"=enum."Move Gantry to Position", "Data"=variant}, error in (no error)=w266) -> (queue out=w263:refnum<queue>, error out=w265:errorcluster)  [unwired: 1 in, 1 out]
      }
      frame "Move Gantry to Position" {
        w283 = 60  # Timeout
        # "When gantry moves all data becomes invalid"
        n81 = flat-sequence {
          tunnel: w281 -> [w296]
          tunnel: [w296] -> w280
          frame #0 {
            "Gantry Moving Message" <- "Gantry Moving" ("Gantry Moving Message")
          }
        }
        n82 = Unbundle By Name(w294) -> ("Configuration.Gantry TCP address:port"=w293:string, "Configuration.X-Position"=w287:dbl, "Configuration.Y-Position"=w286:dbl, "Configuration.Z-Position"=w285:dbl)
        n83 = property on="Next" class="Bool"(error in=w281, "DisabledEnum"=T5."Disabled and Grayed Out" ("Disabled")) -> (error out=w279:errorcluster)  [unwired: 1 in, 1 out]
        n84 = Bundle By Name(cluster=T3 {"Gantry Accel/Decel"=5.0, "Gantry Velocity"=5.0, "X-Position"=0.0, "Y-Position"=0.0, "Z-Position"=0.0} ("Gantry Move Data"), "X-Position"=w287, "Y-Position"=w286, "Z-Position"=w285) -> (w284:T3)
        n85 = Merge Errors(w279, w280) -> (w278:errorcluster)
        n86 = call "Motion_Move Gantry To Position.vi"("Timeout sec (-1 = No timeout)"=w283, "error in"=w278, "Gantry Move Data"=w284, "TCP address:port"=w293) -> ("error out"=w292:errorcluster)  [unwired: 6 in, 1 out]
        n87 = Enqueue Element(queue=w291, element=cluster{"State":T2, "Data":variant} {"State"=enum."Display Attenuation Tab", "Data"=variant}, error in (no error)=w292) -> (queue out=w290:refnum<queue>, error out=w277:errorcluster)  [unwired: 1 in, 1 out]
        n88 = property on="Gantry Moving Message" class="Str"(error in=w277, "Val(Sgnl)"="") -> (error out=w276:errorcluster)  [unwired: 1 in, 1 out]
      }
      frame "Display Attenuation Tab" {
        n89 = property on="Main Tab Control" class="TabCtl (strict)"(error in=w318, "Val(Sgnl)"=T1."Attenuation Tab" ("Value (Signaling)")) -> (error out=w314:errorcluster)  [unwired: 1 in, 1 out]
        n90 = call "Set Button Enable States.vi"("error in (no error)"=w314, "Button States"=T6 {"Prev Button"={"Visible"=TRUE, "Enable"=enum."Enabled"}, "Next Button"={"Visible"=TRUE, "Enable"=enum."Disabled and Grayed Out"}, "Stop Button"={"Visible"=FALSE, "Enable"=enum."Enabled"}}, "queue in"=w315) -> ("error out"=w317:errorcluster, "queue out"=w316:refnum<queue>)  [unwired: 7 in]
        n91 = call "Set Next Action.vi"("Action"=RF_Characterization_States."Display Power Tab", "error in (no error)"=w317, "queue in"=w316) -> ("error out"=w311:errorcluster, "queue out"=w312:refnum<queue>)  [unwired: 7 in]
        n92 = call "Set Prev Action.vi"("Action"=RF_Characterization_States."Display Configuration Tab", "error in (no error)"=w311, "queue in"=w312) -> ("error out"=w300:errorcluster, "queue out"=w301:refnum<queue>)  [unwired: 7 in]
        n93 = call "Set Stop Action.vi"("Action"=RF_Characterization_States."Check Attenuation Results", "error in (no error)"=w300, "queue in"=w301) -> ("error out"=w297:errorcluster, "queue out"=w298:refnum<queue>)  [unwired: 7 in]
        n94 = Enqueue Element(queue=w298, element=cluster{"State":T2, "Data":variant} {"State"=enum."Check Attenuation Config", "Data"=variant}, error in (no error)=w297) -> (queue out=w304:refnum<queue>, error out=w308:errorcluster)  [unwired: 1 in, 1 out]
        n95 = Enqueue Element(queue=w304, element=cluster{"State":T2, "Data":variant} {"State"=enum."Check Attenuation Results", "Data"=variant}, error in (no error)=w308) -> (queue out=w303:refnum<queue>, error out=w305:errorcluster)  [unwired: 1 in, 1 out]
      }
      frame "Check Attenuation Config" {
        n96 = Unbundle("Attenuation Range") -> (w326:dbl, w325:dbl)
        n97 = Less?(x=w326, y=w325) -> (x < y?=w324:bool)
        n98 = case shown="True" w324 {
          tunnel: "Attenuation Increment" -> [_ w360]
          tunnel: "Attenuation Samples" -> [_ w359]
          tunnel: w329 -> [w343 w358]
          tunnel: [w343 w357] -> w328
          tunnel: "Attenuation Range" -> [_ w356]
          tunnel: w323 -> [w341 w355]
          tunnel: w322 -> [w334 w346]
          tunnel: [w341 w355] -> w321
          tunnel: [w340 w351] -> w320
          frame False {
            w337 = u32 14417920
            n99 = property on="Attenuation Range" class="Slide (strict)"(error in=w334) -> (error out=w333:errorcluster, "Active Slider"=w332:i32)  [unwired: 1 in, 1 out]
            n100 = property on="Attenuation Range" class="Slide (strict)"(error in=w333, "FGColor"=w337, "Active Slider"=0, "Fill Color"=w337, "Active Slider"=1, "Fill Color"=w337, "Active Slider"=w332) -> (error out=w338:errorcluster)  [unwired: 1 in, 1 out]
            n101 = property on="Start Attenuation Test" class="Bool"(error in=w334, "DisabledEnum"=T5."Disabled and Grayed Out" ("Disabled")) -> (error out=w339:errorcluster)  [unwired: 1 in, 1 out]
            n102 = Merge Errors(w338, w339) -> (w340:errorcluster)
          }
          frame True {
            w348 = u32 16860
            n103 = Bundle By Name(cluster=w358, "Attenuation Config.Range"=w356, "Attenuation Config.Increment"=w360, "Attenuation Config.Samples"=w359) -> (w357:T4)
            n104 = property on="Attenuation Range" class="Slide (strict)"(error in=w346) -> (error out=w345:errorcluster, "Active Slider"=w344:i32)  [unwired: 1 in, 1 out]
            n105 = property on="Start Attenuation Test" class="Bool"(error in=w346, "DisabledEnum"=T5."Enabled" ("Disabled")) -> (error out=w352:errorcluster)  [unwired: 1 in, 1 out]
            n106 = property on="Attenuation Range" class="Slide (strict)"(error in=w345, "FGColor"=u32 7171459, "Active Slider"=0, "Fill Color"=w348, "Active Slider"=1, "Fill Color"=w348, "Active Slider"=w344) -> (error out=w353:errorcluster)  [unwired: 1 in, 1 out]
            n107 = Merge Errors(w353, w352) -> (w351:errorcluster)
          }
        }
      }
      frame "Start Attenuation Test" {
        n108 = Unbundle By Name(w385) -> ("Attenuation Config.Range"=w393:cluster{dbl, dbl}, "Attenuation Config.Increment"=w392:dbl, "Attenuation Config.Samples"=w391:i32, "Configuration.MICS ID"=w390:u32, "Configuration.MICS Dongle Port"=w389:refnum<visa-resource-name>)
        n109 = property on="Attenuation Graph" class="XYGraph (strict)"(error in=w361, "Active Cursor"=u32 0, "Cursor.Visible"=FALSE) -> (error out=w371:errorcluster)  [unwired: 1 in, 1 out]
        n110 = property on="Start Attenuation Test" class="Bool"(error in=w361, "DisabledEnum"=T5."Disabled and Grayed Out" ("Disabled")) -> (error out=w368:errorcluster)  [unwired: 1 in, 1 out]
        n111 = Merge Errors(w371, w368) -> (w370:errorcluster)
        n112 = Unbundle(w393) -> (w380:dbl, w379:dbl)
        n113 = Bundle(w380, w379, "Increment"=w392) -> (w398:cluster{dbl, dbl, "Increment":dbl})  [unwired: 1 in]
        n114 = Increment(x=w379) -> (x+1=w377:dbl)
        n115 = call "Init MICS.vi"("TARGET MICS ID"=w390, "error in (no error)"=w370, "VISA Resource Name"=w389) -> ("error out"=w387:errorcluster, "dup VISA Resource Name"=w388:refnum<visa-resource-name>)  [unwired: 7 in]
        n116 = Decrement(x=w380) -> (x-1=w378:dbl)
        n117 = call "Range With Increment.vi"("Range"=w398) -> ("Output Array"=w397:dbl[])
        n118 = property on="Attenuation Graph" class="XYGraph (strict)"("XScale.Minimum"=w378, "XScale.Maximum"=w377) -> ()  [unwired: 2 in, 2 out]
        n119 = for {
          tunnel: w388 -> [w416]
          tunnel: w387 -> [w403]
          shift-right: [w413] -> w386
          shift-left: cluster{dbl, dbl}[] [] ("XY Graph") -> [w415]
          tunnel: [w400] -> w396
          tunnel: [w412] -> w395
          tunnel: w397 -> [w410] mode=indexing
          tunnel: w391 -> [w409]
          tunnel: w362 -> [w407]
          tunnel: [w406] -> w375
          stop <- w402 stop-if-true
          n120 = call "Sample MICS Connection Attempts.vi"("MICS Power Setting (0x1F)"=u8 63 ("MICS Power"), "error in"=w403, "Attenuation dB"=w410, "Samples (1)"=w409, "MICS Resource Name"=w416) -> ("error out"=w401:errorcluster, "Percent Successful"=w411:dbl, "MICS Resource Name out"=w412:refnum<visa-resource-name>)  [unwired: 3 in, 1 out]
          n121 = call "Check If Stopped.vi"("error in (no error)"=w403, "queue in"=w407) -> ("error out"=w399:errorcluster, "Stopped?"=w404:bool, "queue out"=w406:refnum<queue>)  [unwired: 7 in]
          n122 = Bundle(w410, "Percent Successful"=w411) -> (w414:cluster{dbl, "Percent Successful":dbl})  [unwired: 1 in]
          n123 = Merge Errors(w401, w399) -> (w400:errorcluster)
          n124 = Build Array (concatenate)(w415, w414) -> (w413:cluster{dbl, "Percent Successful":dbl}[])
          "Attenuation Graph" <- w413
          n125 = Unbundle By Name(w400) -> ("status"=w405:bool)
          n126 = Or(x=w405, y=w404) -> (x .or. y?=w402:bool)
        }
        n127 = VISA Close(VISA resource name=w395, error in (no error)=w396) -> (error out=w366:errorcluster)
        n128 = Bundle By Name(cluster=w385, "Attenuation Results"=w386) -> (w384:T4)
        n129 = property on="Start Attenuation Test" class="Bool"(error in=w366, "DisabledEnum"=T5."Enabled" ("Disabled")) -> (error out=w364:errorcluster)  [unwired: 1 in, 1 out]
        n130 = call "Set Button Enable States.vi"("error in (no error)"=w366, "Button States"=T6 {"Prev Button"={"Visible"=TRUE, "Enable"=enum."Enabled"}, "Next Button"={"Visible"=TRUE, "Enable"=enum."Disabled and Grayed Out"}, "Stop Button"={"Visible"=FALSE, "Enable"=enum."Enabled"}}, "queue in"=w375) -> ("error out"=w365:errorcluster, "queue out"=w374:refnum<queue>)  [unwired: 7 in]
        n131 = Merge Errors(w365, w364) -> (w363:errorcluster)
        n132 = Enqueue Element(queue=w374, element=cluster{"State":T2, "Data":variant} {"State"=enum."Check Attenuation Results", "Data"=variant}, error in (no error)=w363) -> (queue out=w382:refnum<queue>, error out=w383:errorcluster)  [unwired: 1 in, 1 out]
      }
      frame "Check Attenuation Results" {
        n133 = Unbundle By Name(w419) -> ("Attenuation Results"=w420:cluster{dbl, dbl}[])
        n134 = Array Size(array=w420) -> (size(s)=w426:i32)
        n135 = Greater Than 0?(x=w426) -> (x > 0?=w425:bool)
        n136 = case shown="False" w425 {
          tunnel: w424 -> [w434 w447]
          tunnel: w423 -> [w431 w444]
          tunnel: [w432 w445] -> w422
          tunnel: [w429 w442] -> w421
          tunnel: w420 -> [_ w440]
          tunnel: [nan w437] -> w417
          frame False {
            # "No results available - do not allow movement to next step"
            n137 = property on="Attenuation Graph" class="XYGraph (strict)"(error in=w431, "Active Cursor"=u32 0, "Cursor.Visible"=FALSE) -> (error out=w428:errorcluster)  [unwired: 1 in, 1 out]
            n138 = call "Set Button Enable States.vi"("error in (no error)"=w431, "Button States"=T6 {"Prev Button"={"Visible"=TRUE, "Enable"=enum."Enabled"}, "Next Button"={"Visible"=TRUE, "Enable"=enum."Disabled and Grayed Out"}, "Stop Button"={"Visible"=FALSE, "Enable"=enum."Enabled"}}, "queue in"=w434) -> ("error out"=w430:errorcluster, "queue out"=w432:refnum<queue>)  [unwired: 7 in]
            n139 = Merge Errors(w428, w430) -> (w429:errorcluster)
          }
          frame True {
            # "No results available - do not allow movement to next step"
            n140 = property on="Attenuation Graph" class="XYGraph (strict)"(error in=w444, "Active Cursor"=u32 0, "Cursor.Visible"=TRUE) -> (error out=w441:errorcluster, "Cursor.Cursor Index"=w439:i32)  [unwired: 1 in, 1 out]
            n141 = call "Set Button Enable States.vi"("error in (no error)"=w444, "Button States"=T6 {"Prev Button"={"Visible"=TRUE, "Enable"=enum."Enabled"}, "Next Button"={"Visible"=TRUE, "Enable"=enum."Enabled"}, "Stop Button"={"Visible"=FALSE, "Enable"=enum."Enabled"}}, "queue in"=w447) -> ("error out"=w443:errorcluster, "queue out"=w445:refnum<queue>)  [unwired: 7 in]
            n142 = Index Array(array=w440, index=w439) -> (element=w438:cluster{dbl, dbl})
            n143 = Unbundle(w438) -> (w437:dbl)  [unwired: 1 out]
            n144 = Merge Errors(w441, w443) -> (w442:errorcluster)
          }
        }
        "Attenuation Cutoff (dB)" <- w417
        n145 = Bundle By Name(cluster=w419, "Attenuation Cutoff (dB)"=w417) -> (w418:T4)
      }
      frame "Display Power Tab" {
        n146 = property on="Main Tab Control" class="TabCtl (strict)"(error in=w453, "Val(Sgnl)"=T1."MICS Power Tab" ("Value (Signaling)")) -> (error out=w469:errorcluster)  [unwired: 1 in, 1 out]
        n147 = call "Set Button Enable States.vi"("error in (no error)"=w469, "Button States"=T6 {"Prev Button"={"Visible"=TRUE, "Enable"=enum."Enabled"}, "Next Button"={"Visible"=TRUE, "Enable"=enum."Disabled and Grayed Out"}, "Stop Button"={"Visible"=FALSE, "Enable"=enum."Enabled"}}, "queue in"=w452) -> ("error out"=w471:errorcluster, "queue out"=w470:refnum<queue>)  [unwired: 7 in]
        n148 = call "Set Next Action.vi"("Action"=RF_Characterization_States."Display Mapping Tab", "error in (no error)"=w471, "queue in"=w470) -> ("error out"=w466:errorcluster, "queue out"=w467:refnum<queue>)  [unwired: 7 in]
        n149 = call "Set Prev Action.vi"("Action"=RF_Characterization_States."Display Attenuation Tab", "error in (no error)"=w466, "queue in"=w467) -> ("error out"=w457:errorcluster, "queue out"=w458:refnum<queue>)  [unwired: 7 in]
        n150 = call "Set Stop Action.vi"("Action"=RF_Characterization_States."Check Power Results", "error in (no error)"=w457, "queue in"=w458) -> ("error out"=w454:errorcluster, "queue out"=w455:refnum<queue>)  [unwired: 7 in]
        n151 = Enqueue Element(queue=w455, element=cluster{"State":T2, "Data":variant} {"State"=enum."Check Power Config", "Data"=variant}, error in (no error)=w454) -> (queue out=w460:refnum<queue>, error out=w463:errorcluster)  [unwired: 1 in, 1 out]
        n152 = Enqueue Element(queue=w460, element=cluster{"State":T2, "Data":variant} {"State"=enum."Check Power Results", "Data"=variant}, error in (no error)=w463) -> (queue out=w451:refnum<queue>, error out=w450:errorcluster)  [unwired: 1 in, 1 out]
      }
      frame "Check Power Config" {
        n153 = Unbundle("Power Range") -> (w484:dbl, w483:dbl)
        n154 = Less?(x=w484, y=w483) -> (x < y?=w482:bool)
        n155 = case shown="True" w482 {
          tunnel: "Power Increment" -> [_ w513]
          tunnel: "Power Samples" -> [_ w512]
          tunnel: w474 -> [w496 w511]
          tunnel: [w496 w510] -> w473
          tunnel: "Power Range" -> [_ w509]
          tunnel: w481 -> [w494 w508]
          tunnel: w480 -> [w487 w499]
          tunnel: [w494 w508] -> w479
          tunnel: [w493 w504] -> w478
          frame False {
            w490 = u32 14417920
            n156 = property on="Power Range" class="Slide (strict)"(error in=w487) -> (error out=w486:errorcluster, "Active Slider"=w485:i32)  [unwired: 1 in, 1 out]
            n157 = property on="Power Range" class="Slide (strict)"(error in=w486, "FGColor"=w490, "Active Slider"=0, "Fill Color"=w490, "Active Slider"=1, "Fill Color"=w490, "Active Slider"=w485) -> (error out=w491:errorcluster)  [unwired: 1 in, 1 out]
            n158 = property on="Start Power Test" class="Bool"(error in=w487, "DisabledEnum"=T5."Disabled and Grayed Out" ("Disabled")) -> (error out=w492:errorcluster)  [unwired: 1 in, 1 out]
            n159 = Merge Errors(w491, w492) -> (w493:errorcluster)
          }
          frame True {
            w501 = u32 16860
            n160 = Bundle By Name(cluster=w511, "Power Config.Range"=w509, "Power Config.Increment"=w513, "Power Config.Samples"=w512) -> (w510:T4)
            n161 = property on="Power Range" class="Slide (strict)"(error in=w499) -> (error out=w498:errorcluster, "Active Slider"=w497:i32)  [unwired: 1 in, 1 out]
            n162 = property on="Start Power Test" class="Bool"(error in=w499, "DisabledEnum"=T5."Enabled" ("Disabled")) -> (error out=w505:errorcluster)  [unwired: 1 in, 1 out]
            n163 = property on="Power Range" class="Slide (strict)"(error in=w498, "FGColor"=u32 7171459, "Active Slider"=0, "Fill Color"=w501, "Active Slider"=1, "Fill Color"=w501, "Active Slider"=w497) -> (error out=w506:errorcluster)  [unwired: 1 in, 1 out]
            n164 = Merge Errors(w506, w505) -> (w504:errorcluster)
          }
        }
      }
      frame "Start Power Test" {
        n165 = Unbundle By Name(w540) -> ("Power Config.Range"=w547:cluster{dbl, dbl}, "Power Config.Increment"=w514:dbl, "Power Config.Samples"=w546:i32, "Attenuation Cutoff (dB)"=w515:dbl, "Configuration.MICS ID"=w545:u32, "Configuration.MICS Dongle Port"=w544:refnum<visa-resource-name>)
        n166 = property on="MICS Power Graph" class="XYGraph (strict)"(error in=w516, "Active Cursor"=u32 0, "Cursor.Visible"=FALSE) -> (error out=w526:errorcluster)  [unwired: 1 in, 1 out]
        n167 = property on="Start Power Test" class="Bool"(error in=w516, "DisabledEnum"=T5."Disabled and Grayed Out" ("Disabled")) -> (error out=w523:errorcluster)  [unwired: 1 in, 1 out]
        n168 = Merge Errors(w526, w523) -> (w525:errorcluster)
        n169 = Unbundle(w547) -> (w535:dbl, w534:dbl)
        n170 = Bundle(w535, w534, "Increment"=w514) -> (w552:cluster{dbl, dbl, "Increment":dbl})  [unwired: 1 in]
        n171 = Increment(x=w534) -> (x+1=w532:dbl)
        n172 = call "Init MICS.vi"("TARGET MICS ID"=w545, "error in (no error)"=w525, "VISA Resource Name"=w544) -> ("error out"=w542:errorcluster, "dup VISA Resource Name"=w543:refnum<visa-resource-name>)  [unwired: 7 in]
        n173 = Decrement(x=w535) -> (x-1=w533:dbl)
        n174 = call "Range With Increment.vi"("Range"=w552) -> ("Output Array"=w551:dbl[])
        n175 = property on="MICS Power Graph" class="XYGraph (strict)"("XScale.Minimum"=w533, "XScale.Maximum"=w532) -> ()  [unwired: 2 in, 2 out]
        n176 = for {
          tunnel: w543 -> [w571]
          tunnel: w542 -> [w561]
          shift-right: [w556] -> w541
          shift-left: cluster{dbl, dbl}[] [] ("XY Graph") -> [w570]
          tunnel: [w558] -> w550
          tunnel: [w568] -> w549
          tunnel: w551 -> [w555] mode=indexing
          tunnel: w546 -> [w566]
          tunnel: w517 -> [w565]
          tunnel: [w564] -> w530
          tunnel: w515 -> [w553]
          stop <- w560 stop-if-true
          n177 = To Unsigned Byte Integer(number=w555) -> (unsigned 8bit integer=w554:u8)
          n178 = call "Sample MICS Connection Attempts.vi"("MICS Power Setting (0x1F)"=w554, "error in"=w561, "Attenuation dB"=w553, "Samples (1)"=w566, "MICS Resource Name"=w571) -> ("error out"=w559:errorcluster, "Percent Successful"=w567:dbl, "MICS Resource Name out"=w568:refnum<visa-resource-name>)  [unwired: 3 in, 1 out]
          n179 = call "Check If Stopped.vi"("error in (no error)"=w561, "queue in"=w565) -> ("error out"=w557:errorcluster, "Stopped?"=w562:bool, "queue out"=w564:refnum<queue>)  [unwired: 7 in]
          n180 = Bundle(w555, "Percent Successful"=w567) -> (w569:cluster{dbl, "Percent Successful":dbl})  [unwired: 1 in]
          n181 = Merge Errors(w559, w557) -> (w558:errorcluster)
          n182 = Build Array (concatenate)(w570, w569) -> (w556:cluster{dbl, "Percent Successful":dbl}[])
          "MICS Power Graph" <- w556
          n183 = Unbundle By Name(w558) -> ("status"=w563:bool)
          n184 = Or(x=w563, y=w562) -> (x .or. y?=w560:bool)
        }
        n185 = VISA Close(VISA resource name=w549, error in (no error)=w550) -> (error out=w521:errorcluster)
        n186 = Bundle By Name(cluster=w540, "Power Results"=w541) -> (w539:T4)
        n187 = property on="Start Power Test" class="Bool"(error in=w521, "DisabledEnum"=T5."Enabled" ("Disabled")) -> (error out=w519:errorcluster)  [unwired: 1 in, 1 out]
        n188 = call "Set Button Enable States.vi"("error in (no error)"=w521, "Button States"=T6 {"Prev Button"={"Visible"=TRUE, "Enable"=enum."Enabled"}, "Next Button"={"Visible"=TRUE, "Enable"=enum."Disabled and Grayed Out"}, "Stop Button"={"Visible"=FALSE, "Enable"=enum."Enabled"}}, "queue in"=w530) -> ("error out"=w520:errorcluster, "queue out"=w529:refnum<queue>)  [unwired: 7 in]
        n189 = Merge Errors(w520, w519) -> (w518:errorcluster)
        n190 = Enqueue Element(queue=w529, element=cluster{"State":T2, "Data":variant} {"State"=enum."Check Power Results", "Data"=variant}, error in (no error)=w518) -> (queue out=w537:refnum<queue>, error out=w538:errorcluster)  [unwired: 1 in, 1 out]
      }
      frame "Check Power Results" {
        n191 = Unbundle By Name(w574) -> ("Power Results"=w575:cluster{dbl, dbl}[])
        n192 = Array Size(array=w575) -> (size(s)=w581:i32)
        n193 = Greater Than 0?(x=w581) -> (x > 0?=w580:bool)
        n194 = case shown="False" w580 {
          tunnel: w579 -> [w589 w603]
          tunnel: w578 -> [w586 w600]
          tunnel: [w587 w601] -> w577
          tunnel: [w584 w598] -> w576
          tunnel: w575 -> [_ w596]
          tunnel: [0 w592] -> w572
          frame False {
            # "No results available - do not allow movement to next step"
            n195 = property on="MICS Power Graph" class="XYGraph (strict)"(error in=w586, "Active Cursor"=u32 0, "Cursor.Visible"=FALSE) -> (error out=w583:errorcluster)  [unwired: 1 in, 1 out]
            n196 = call "Set Button Enable States.vi"("error in (no error)"=w586, "Button States"=T6 {"Prev Button"={"Visible"=TRUE, "Enable"=enum."Enabled"}, "Next Button"={"Visible"=TRUE, "Enable"=enum."Disabled and Grayed Out"}, "Stop Button"={"Visible"=FALSE, "Enable"=enum."Enabled"}}, "queue in"=w589) -> ("error out"=w585:errorcluster, "queue out"=w587:refnum<queue>)  [unwired: 7 in]
            n197 = Merge Errors(w583, w585) -> (w584:errorcluster)
          }
          frame True {
            # "No results available - do not allow movement to next step"
            n198 = property on="MICS Power Graph" class="XYGraph (strict)"(error in=w600, "Active Cursor"=u32 0, "Cursor.Visible"=TRUE) -> (error out=w597:errorcluster, "Cursor.Cursor Index"=w595:i32)  [unwired: 1 in, 1 out]
            n199 = call "Set Button Enable States.vi"("error in (no error)"=w600, "Button States"=T6 {"Prev Button"={"Visible"=TRUE, "Enable"=enum."Enabled"}, "Next Button"={"Visible"=TRUE, "Enable"=enum."Enabled"}, "Stop Button"={"Visible"=FALSE, "Enable"=enum."Enabled"}}, "queue in"=w603) -> ("error out"=w599:errorcluster, "queue out"=w601:refnum<queue>)  [unwired: 7 in]
            n200 = Index Array(array=w596, index=w595) -> (element=w594:cluster{dbl, dbl})
            n201 = Unbundle(w594) -> (w593:dbl)  [unwired: 1 out]
            n202 = Merge Errors(w597, w599) -> (w598:errorcluster)
            n203 = To Long Integer(number=w593) -> (32bit integer=w592:i32)
          }
        }
        "Power Cutoff" <- w572
        n204 = Bundle By Name(cluster=w574, "Power Cutoff"=w572) -> (w573:T4)
      }
      frame "Display Mapping Tab" {
        n205 = property on="Main Tab Control" class="TabCtl (strict)"(error in=w608, "Val(Sgnl)"=T1."RF Mapping Tab" ("Value (Signaling)")) -> (error out=w625:errorcluster)  [unwired: 1 in, 1 out]
        n206 = call "Set Button Enable States.vi"("error in (no error)"=w625, "Button States"=T6 {"Prev Button"={"Visible"=TRUE, "Enable"=enum."Enabled"}, "Next Button"={"Visible"=TRUE, "Enable"=enum."Disabled and Grayed Out"}, "Stop Button"={"Visible"=FALSE, "Enable"=enum."Enabled"}}, "queue in"=w609) -> ("error out"=w627:errorcluster, "queue out"=w626:refnum<queue>)  [unwired: 7 in]
        n207 = call "Set Next Action.vi"("Action"=RF_Characterization_States."Display Report Tab", "error in (no error)"=w627, "queue in"=w626) -> ("error out"=w622:errorcluster, "queue out"=w623:refnum<queue>)  [unwired: 7 in]
        n208 = call "Set Prev Action.vi"("Action"=RF_Characterization_States."Display Power Tab", "error in (no error)"=w622, "queue in"=w623) -> ("error out"=w613:errorcluster, "queue out"=w614:refnum<queue>)  [unwired: 7 in]
        n209 = call "Set Stop Action.vi"("Action"=RF_Characterization_States."Finish Mapping Test", "error in (no error)"=w613, "queue in"=w614) -> ("error out"=w610:errorcluster, "queue out"=w611:refnum<queue>)  [unwired: 7 in]
        n210 = Enqueue Element(queue=w611, element=cluster{"State":T2, "Data":variant} {"State"=enum."Check Mapping Config", "Data"=variant}, error in (no error)=w610) -> (queue out=w616:refnum<queue>, error out=w619:errorcluster)  [unwired: 1 in, 1 out]
        n211 = Enqueue Element(queue=w616, element=cluster{"State":T2, "Data":variant} {"State"=enum."Check Mapping Results", "Data"=variant}, error in (no error)=w619) -> (queue out=w607:refnum<queue>, error out=w606:errorcluster)  [unwired: 1 in, 1 out]
      }
      frame "Check Mapping Config" {
      }
      frame "Start Mapping Test" {
        n212 = control-ref of="RF Mapping Graph"() -> (w665:refnum<vi>)
        n213 = Unbundle By Name(w654) -> ("Configuration.MICS ID"=w656:u32, "Configuration.MICS Dongle Port"=w657:refnum<visa-resource-name>, "Configuration.Gantry TCP address:port"=w652:string)
        n214 = property on="Start Power Test" class="Bool"(error in=w650, "DisabledEnum"=T5."Disabled and Grayed Out" ("Disabled")) -> (error out=w649:errorcluster)  [unwired: 1 in, 1 out]
        n215 = call "Generate Sampling Positions.vi"("Gantry Accel/Decel"=5.0, "Gantry Velocity"=5.0, "Z Range"="Z Range", "Y Range"="Y Range", "X Range"="X Range") -> ("Dimensions"=w664:i32[], "Indices"=w660:cluster{i32, i32, i32}[], "Output"=w661:T3[])  [unwired: 4 in]
        n216 = call "Scale Intensity Plot.vi"("Dimensions"=w664, "Y Range"="Y Range", "X Range"="X Range", "IntGraph Refnum"=w665) -> ()  [unwired: 6 in, 2 out]
        n217 = Index Array(array=w664) -> (element #1=w669:i32, element #2=w668:i32, element #3=w667:i32)  [unwired: 3 in]
        n218 = Initialize Array(nan ("element"), w669, w668, w667) -> (w659:dbl[][][])
        n219 = call "Init MICS.vi"("TARGET MICS ID"=w656, "error in (no error)"=w649, "VISA Resource Name"=w657) -> ("error out"=w655:errorcluster, "dup VISA Resource Name"=w653:refnum<visa-resource-name>)  [unwired: 7 in]
        n220 = call "Motion_Initialize.vi"("error in (no error)"=w655, "TCP address:port (192.168.0.3:502)"=w652) -> ("error out"=w635:errorcluster, "connection ID"=w633:refnum<k5>)  [unwired: 8 in]
        n221 = Bundle By Name(cluster=w654, "Mapping Config.Samples"="Mapping Samples", "Mapping Config.X Range"="X Range", "Mapping Config.Y Range"="Y Range", "Mapping Config.Z Range"="Z Range", "Mapping Config.Positions"=w661, "Mapping Config.Indices"=w660, "Mapping Results"=w659, "Refnums.MICS Refnum"=w653, "Refnums.Motion Refnum"=w633) -> (w636:T4)
        n222 = call "Motion_Gantry Enable.vi"("error in (no error)"=w635, "Enable? (T)"=TRUE, "TCP Connection Refnum in"=w633) -> ("error out"=w634:errorcluster)  [unwired: 7 in, 1 out]
        n223 = Unbundle By Name(w636) -> ("Mapping Config.Z Range.Increment"=w637:dbl, "Mapping Config.Z Range.Max"=w638:dbl, "Mapping Config.Z Range.Min"=w639:dbl)
        n224 = property on="Z-Layer" class="Slide (strict)"(error in=w634, "Increment"=w637, "Maximum"=w638, "Minimum"=w639) -> (error out=w640:errorcluster)  [unwired: 1 in, 1 out]
        n225 = call "Set Button Enable States.vi"("error in (no error)"=w640, "Button States"=T6 {"Prev Button"={"Visible"=TRUE, "Enable"=enum."Disabled and Grayed Out"}, "Next Button"={"Visible"=TRUE, "Enable"=enum."Disabled and Grayed Out"}, "Stop Button"={"Visible"=TRUE, "Enable"=enum."Enabled"}}, "queue in"=w642) -> ("error out"=w645:errorcluster, "queue out"=w646:refnum<queue>)  [unwired: 7 in]
        n226 = Enqueue Element(queue=w646, element=cluster{"State":T2, "Data":variant} {"State"=enum."Take Mapping Sample", "Data"=variant}, error in (no error)=w645) -> (queue out=w644:refnum<queue>, error out=w643:errorcluster)  [unwired: 1 in, 1 out]
      }
      frame "Take Mapping Sample" {
        w703 = 0.1  # Tolerance
        n227 = Unbundle By Name(w709) -> ("Mapping Index"=w696:i32, "Mapping Results"=w714:dbl[][][], "Mapping Config.Indices"=w711:cluster{i32, i32, i32}[], "Mapping Index"=w701:i32, "Power Cutoff"=w700:u8, "Refnums.MICS Refnum"=w699:refnum<visa-resource-name>, "Mapping Config.Samples"=w698:i32, "Attenuation Cutoff (dB)"=w697:dbl, "Mapping Config.Positions"=w692:T3[], "Mapping Index"=w702:i32, "Refnums.Motion Refnum"=w713:refnum<k5>)
        n228 = Index Array(array=w692, index=w702) -> (element=w672:T3)
        n229 = Index Array(array=w711, index=w701) -> (element=w712:cluster{i32, i32, i32})
        n230 = Array Size(array=w692) -> (size(s)=w690:i32)
        n231 = call "Motion_Gantry Move.vi"("error in (no error)"=w715, "Gantry Move Data"=w672, "TCP Connection Refnum in"=w713) -> ("error out"=w681:errorcluster, "TCP Connection Refnum (dup)"=w683:refnum<k5>)  [unwired: 7 in]
        n232 = call "Motion_Wait for Gantry Move.vi"("error in (no error)"=w681, "Timeout sec (-1 = No timeout)"=60, "TCP Connection Refnum in"=w683) -> ("error out"=w680:errorcluster, "Timed Out?"=w676:bool, "TCP Connection Refnum (dup)"=w682:refnum<k5>)  [unwired: 5 in, 1 out]
        n233 = call "Motion_Gantry Check Position.vi"("Tolerance (0.1)"=w703, "error in (no error)"=w680, "Gantry Move Data"=w672, "TCP Connection Refnum"=w682) -> ("error out"=w674:errorcluster, "In Position?"=w678:bool)  [unwired: 5 in, 1 out]
        n234 = Not(x=w678) -> (.not. x?=w677:bool)
        n235 = Or(x=w676, y=w677) -> (x .or. y?=w679:bool)
        n236 = Select(t=errorcluster {"status"=TRUE, "code"=-1, "source"="Gantry not in position"} ("error out"), s=w679, f=w674) -> (s? t:f=w673:errorcluster)
        n237 = call "Sample MICS Connection Attempts.vi"("MICS Power Setting (0x1F)"=w700, "error in"=w673, "Attenuation dB"=w697, "Samples (1)"=w698, "MICS Resource Name"=w699) -> ("error out"=w695:errorcluster, "Percent Successful"=w704:dbl)  [unwired: 3 in, 2 out]
        n238 = Unbundle(w712) -> (w707:i32, w706:i32, w705:i32)
        n239 = Replace Array Subset(array=w714, new element=w704, index (dim 0)=w707, index (dim 1)=w706, index (dim 2)=w705) -> (w710:dbl[][][])
        n240 = Increment(x=w696) -> (x+1=w691:i32)
        n241 = Greater Or Equal?(x=w691, y=w690) -> (x >= y?=w689:bool)
        n242 = Bundle By Name(cluster=w709, "Mapping Index"=w691, "Mapping Results"=w710) -> (w708:T4)
        n243 = Enqueue Element(queue=w687, element=cluster{"State":T2, "Data":variant} {"State"=enum."Check Mapping Results", "Data"=variant}, error in (no error)=w695) -> (queue out=w686:refnum<queue>, error out=w688:errorcluster)  [unwired: 1 in, 1 out]
        n244 = case shown="True" w689 {
          tunnel: w688 -> [w720 w721]
          tunnel: [w719 w725] -> w694
          tunnel: w686 -> [w718 w722]
          tunnel: [w717 w724] -> w693
          frame True {
            n245 = Enqueue Element(queue=w718, element=cluster{"State":T2, "Data":variant} {"State"=enum."Finish Mapping Test", "Data"=variant}, error in (no error)=w720) -> (queue out=w717:refnum<queue>, error out=w719:errorcluster)  [unwired: 1 in, 1 out]
          }
          frame False {
            n246 = Enqueue Element(queue=w722, element=cluster{"State":T2, "Data":variant} {"State"=enum."Take Mapping Sample", "Data"=variant}, error in (no error)=w721) -> (queue out=w724:refnum<queue>, error out=w725:errorcluster)  [unwired: 1 in, 1 out]
          }
        }
      }
      frame "Finish Mapping Test" {
        n247 = Unbundle By Name(w737) -> ("Refnums.MICS Refnum"=w739:refnum<visa-resource-name>, "Refnums.Motion Refnum"=w738:refnum<k5>)
        n248 = property on="Start Power Test" class="Bool"(error in=w735, "DisabledEnum"=T5."Enabled" ("Disabled")) -> (error out=w734:errorcluster)  [unwired: 1 in, 1 out]
        n249 = VISA Close(VISA resource name=w739, error in (no error)=w735) -> (error out=w741:errorcluster)
        n250 = call "Motion_Close.vi"("error in (no error)"=w735, "connection ID"=w738) -> ("error out"=w740:errorcluster)  [unwired: 9 in]
        n251 = Merge Errors(w741, w740, w734) -> (w731:errorcluster)
        n252 = call "Set Button Enable States.vi"("error in (no error)"=w731, "Button States"=T6 {"Prev Button"={"Visible"=TRUE, "Enable"=enum."Enabled"}, "Next Button"={"Visible"=TRUE, "Enable"=enum."Enabled"}, "Stop Button"={"Visible"=FALSE, "Enable"=enum."Enabled"}}, "queue in"=w732) -> ("error out"=w729:errorcluster, "queue out"=w728:refnum<queue>)  [unwired: 7 in]
        n253 = Enqueue Element(queue=w728, element=cluster{"State":T2, "Data":variant} {"State"=enum."Check Mapping Results", "Data"=variant}, error in (no error)=w729) -> (queue out=w727:refnum<queue>, error out=w726:errorcluster)  [unwired: 1 in, 1 out]
      }
      frame "Check Mapping Results" {
        n254 = Unbundle By Name(w749) -> ("Mapping Results"=w745:dbl[][][], "Mapping Config.Z Range"=w743:cluster{"Min":dbl, "Max":dbl, "Increment":dbl})
        n255 = call "Range With Increment.vi"("Range"=w743) -> ("Output Array"=w742:dbl[])
        n256 = Threshold 1D Array(2:"Z-Layer", 3:w742) -> (0:w748:dbl)  [unwired: 1 in]
        n257 = Round To Nearest(number=w748) -> (nearest integer value=w747:dbl)
        n258 = To Long Integer(number=w747) -> (32bit integer=w746:i32)
        n259 = Index Array(array=w745, index (dim 2)=w746) -> (element=→"RF Mapping Graph":dbl[][])  [unwired: 2 in]
      }
      frame "Display Report Tab" {
        w769 = RF_Characterization_States."Error" ("Action")
        n260 = property on="Main Tab Control" class="TabCtl (strict)"(error in=w770, "Val(Sgnl)"=T1."Create Report" ("Value (Signaling)")) -> (error out=w759:errorcluster)  [unwired: 1 in, 1 out]
        n261 = call "Set Button Enable States.vi"("error in (no error)"=w759, "Button States"=T6 {"Prev Button"={"Visible"=TRUE, "Enable"=enum."Enabled"}, "Next Button"={"Visible"=FALSE, "Enable"=enum."Enabled"}, "Stop Button"={"Visible"=FALSE, "Enable"=enum."Enabled"}}, "queue in"=w760) -> ("error out"=w768:errorcluster, "queue out"=w767:refnum<queue>)  [unwired: 7 in]
        n262 = call "Set Next Action.vi"("Action"=w769, "error in (no error)"=w768, "queue in"=w767) -> ("error out"=w764:errorcluster, "queue out"=w765:refnum<queue>)  [unwired: 7 in]
        n263 = call "Set Prev Action.vi"("Action"=RF_Characterization_States."Display Mapping Tab", "error in (no error)"=w764, "queue in"=w765) -> ("error out"=w761:errorcluster, "queue out"=w762:refnum<queue>)  [unwired: 7 in]
        n264 = call "Set Stop Action.vi"("Action"=w769, "error in (no error)"=w761, "queue in"=w762) -> ("error out"=w758:errorcluster, "queue out"=w755:refnum<queue>)  [unwired: 7 in]
        n265 = Enqueue Element(queue=w755, element=cluster{"State":T2, "Data":variant} {"State"=enum."Generate Report", "Data"=variant}, error in (no error)=w758) -> (queue out=w754:refnum<queue>, error out=w756:errorcluster)  [unwired: 1 in, 1 out]
      }
      frame "Generate Report" {
        n266 = Unbundle By Name(w774) -> ("Report"=w775:refnum<class "NI_report.lvclass">)
        n267 = while {
          shift-right: [w786] -> _
          shift-left: Report_Generation_States."Initialize" ("Report Generation States") -> [w788]
          tunnel: w776 -> [w785]
          tunnel: [w783] -> w777
          shift-right: [w782] -> _
          shift-left: w774 -> [w784]
          shift-right: [w780] -> w773
          shift-left: w775 -> [w781]
          stop <- w787 stop-if-true
          n268 = case shown="\"Generate Summary\"" w788 {
            tunnel: [_ _ _ _ _ _ _ TRUE] -> w787
            tunnel: [Report_Generation_States."Generate Header" ("Report Generation States") Report_Generation_States."Generate Summary" ("Report Generation States") Report_Generation_States."Generate Attenuation Section" ("Report Generation States") Report_Generation_States."Generate MICS Power Section" ("Report Generation States") Report_Generation_States."Generate RF Mapping Section 1" ("Report Generation States") Report_Generation_States."Generate RF Mapping Section 2" ("Report Generation States") Report_Generation_States."Show Report in UI" ("Report Generation States") Report_Generation_States."Show Report in UI" ("Report Generation States")] -> w786
            tunnel: w785 -> [w793 w804 w832 w873 w919 w947 w955 w1000]
            tunnel: w784 -> [w797 w806 w810 w850 w896 w940 w966 w1006]
            tunnel: [w791 w800 w808 w862 w908 w926 w958 w998] -> w783
            tunnel: [w797 w806 w810 w850 w896 w940 w966 w1006] -> w782
            tunnel: w781 -> [w796 w803 w829 w856 w902 w946 w956 w999]
            tunnel: [w790 w801 w809 w863 w909 w925 w957 w997] -> w780
            frame "Initialize" {
              # "Dispose previous report (if any) and create new report"
              n269 = call-dynamic "Dispose Report.vi"("report in"=w796, "error in (no error)"=w793) -> ("error out"=w798:errorcluster)  [unwired: 13 in]
              n270 = call <vilib>:"Clear Errors.vi"("error in (no error)"=w798) -> ("error out"=w794:errorcluster)  [unwired: 6 in]
              n271 = Merge Errors(w794, w793) -> (w792:errorcluster)
              n272 = call <vilib>:"New Report.vi"("report type"=T9."HTML", "error in (no error)"=w792) -> ("report out"=w790:refnum<class "NI_report.lvclass">, "error out"=w791:errorcluster)  [unwired: 12 in]
            }
            frame "Generate Header" {
              n273 = call "Report - Add Section Header.vi"("report in"=w803, "Heading Size"=enum16{"h1", "h2", "h3"}."h1", "Heading Text"="RF Mapping Report" ("text"), "error in (no error)"=w804) -> ("report out"=w801:refnum<class "NI_report.lvclass">, "error out"=w800:errorcluster)  [unwired: 10 in]
            }
            frame "Generate Summary" {
              n274 = call-dynamic "Append Horizontal Line to Report.vi"("report in"=w829, "error in (no error)"=w832) -> ("report out"=w827:refnum<class "NI_report.lvclass">, "error out"=w826:errorcluster)  [unwired: 12 in]
              n275 = Unbundle By Name(w810) -> ("Configuration.X-Position"=w822:dbl, "Configuration.Y-Position"=w821:dbl, "Configuration.Z-Position"=w820:dbl)
              n276 = Unbundle By Name(w810) -> ("Configuration.MICS ID"=w817:u32)
              n277 = Format Date/Time String() -> (date/time string=w815:string)  [unwired: 3 in]
              n278 = call "Report - Add Section Header.vi"("report in"=w827, "Heading Size"=enum16{"h1", "h2", "h3"}."h2", "Heading Text"="Summary", "error in (no error)"=w826) -> ("report out"=w824:refnum<class "NI_report.lvclass">, "error out"=w823:errorcluster)  [unwired: 10 in]
              n279 = Number To Decimal String(number=w817) -> (decimal integer string=w816:string)  [unwired: 1 in]
              n280 = Format Into String(format string="(%.3f, %.3f, %.3f)", w822, w821, w820) -> (resulting string=w814:string)  [unwired: 2 in, 1 out]
              n281 = Build Array(w816, w815, w814) -> (w812:string[])
              n282 = Build Array(w812) -> (w811:string[][])
              n283 = Transpose 2D Array(2D array=w811) -> (transposed array=w807:string[][])
              n284 = call-poly <vilib>:"Append Table to Report.vi"("report in"=w824, "row headers"=string[] ["MICS ID", "Completed At", "Gantry Position"] ("column headers"), "text data"=w807, "error in (no error)"=w823) -> ("report out"=w831:refnum<class "NI_report.lvclass">, "error out"=w830:errorcluster)  [unwired: 8 in, 2 out]
              n285 = call-dynamic "New Report Line.vi"("report in"=w831, "error in (no error)"=w830) -> ("report out"=w809:refnum<class "NI_report.lvclass">, "error out"=w808:errorcluster)  [unwired: 12 in]
            }
            frame "Generate Attenuation Section" {
              n286 = call-dynamic "Append Horizontal Line to Report.vi"("report in"=w856, "error in (no error)"=w873) -> ("report out"=w853:refnum<class "NI_report.lvclass">, "error out"=w852:errorcluster)  [unwired: 12 in]
              n287 = Unbundle By Name(w850) -> ("Attenuation Results"=w871:cluster{dbl, dbl}[])
              n288 = Unbundle By Name(w850) -> ("Attenuation Config.Range"=w844:cluster{dbl, dbl}, "Attenuation Config.Increment"=w840:dbl, "Attenuation Config.Samples"=w839:i32)
              n289 = call "Report - Add Section Header.vi"("report in"=w853, "Heading Size"=enum16{"h1", "h2", "h3"}."h2", "Heading Text"="Attenuation Results" ("text"), "error in (no error)"=w852) -> ("report out"=w848:refnum<class "NI_report.lvclass">, "error out"=w847:errorcluster)  [unwired: 10 in]
              n290 = Unbundle(w844) -> (w843:dbl, w842:dbl)
              n291 = for {
                tunnel: w871 -> [w878] mode=indexing
                tunnel: [w876] -> w870 mode=indexing
                tunnel: [w874] -> w869 mode=indexing
                n292 = Unbundle(w878) -> (w877:dbl, w875:dbl)
                n293 = Number To Fractional String(number=w877) -> (F-format string=w876:string)  [unwired: 3 in]
                n294 = Number To Fractional String(number=w875) -> (F-format string=w874:string)  [unwired: 3 in]
              }
              n295 = Format Into String(format string="Range: %.3f to %.3f", w843, w842) -> (resulting string=w836:string)  [unwired: 2 in, 1 out]
              n296 = Format Into String(format string="Increment: %.3f", w840) -> (resulting string=w835:string)  [unwired: 2 in, 1 out]
              n297 = Format Into String(format string="Samples: %d", w839) -> (resulting string=w834:string)  [unwired: 2 in, 1 out]
              n298 = Build Array(w836, w835, w834) -> (w833:string[])
              n299 = Build Array(w870, w869) -> (w868:string[][])
              n300 = Transpose 2D Array(2D array=w868) -> (transposed array=w861:string[][])
              n301 = call-dynamic "Append List to Report.vi"("report in"=w848, "list elements"=w833, "list type (ordered)"=enum16{"unordered", "ordered"}."unordered", "error in (no error)"=w847) -> ("report out"=w846:refnum<class "NI_report.lvclass">, "error out"=w845:errorcluster)  [unwired: 8 in, 2 out]
              n302 = call-poly <vilib>:"Append Table to Report.vi"("report in"=w846, "column headers"=string[] ["Attenuation (dB)", "Percent Success"], "text data"=w861, "error in (no error)"=w845) -> ("report out"=w860:refnum<class "NI_report.lvclass">, "error out"=w858:errorcluster)  [unwired: 8 in, 2 out]
              n303 = control-ref of="Attenuation Graph"() -> (w867:refnum<vi>)
              n304 = call-dynamic "New Report Line.vi"("report in"=w860, "error in (no error)"=w858) -> ("report out"=w859:refnum<class "NI_report.lvclass">, "error out"=w857:errorcluster)  [unwired: 12 in]
              n305 = To More Generic Class(target class=refnum<vi> refnum ("ctrl reference"), reference=w867) -> (generic class reference=w865:refnum<vi>)
              n306 = call-dynamic "Append Control Image to Report.vi"("report in"=w859, "ctrl reference"=w865, "description"="Attenuation Graph", "error in (no error)"=w857) -> ("report out"=w863:refnum<class "NI_report.lvclass">, "error out"=w862:errorcluster)  [unwired: 8 in, 2 out]
            }
            frame "Generate MICS Power Section" {
              n307 = call-dynamic "Append Horizontal Line to Report.vi"("report in"=w902, "error in (no error)"=w919) -> ("report out"=w899:refnum<class "NI_report.lvclass">, "error out"=w898:errorcluster)  [unwired: 12 in]
              n308 = Unbundle By Name(w896) -> ("Power Config.Range"=w890:cluster{dbl, dbl}, "Power Config.Increment"=w886:dbl, "Power Config.Samples"=w885:i32)
              n309 = Unbundle By Name(w896) -> ("Power Results"=w917:cluster{dbl, dbl}[])
              n310 = call "Report - Add Section Header.vi"("report in"=w899, "Heading Size"=enum16{"h1", "h2", "h3"}."h2", "Heading Text"="MICS Power Results" ("text"), "error in (no error)"=w898) -> ("report out"=w894:refnum<class "NI_report.lvclass">, "error out"=w893:errorcluster)  [unwired: 10 in]
              n311 = Unbundle(w890) -> (w889:dbl, w888:dbl)
              n312 = for {
                tunnel: w917 -> [w924] mode=indexing
                tunnel: [w922] -> w916 mode=indexing
                tunnel: [w920] -> w915 mode=indexing
                n313 = Unbundle(w924) -> (w923:dbl, w921:dbl)
                n314 = Number To Fractional String(number=w923) -> (F-format string=w922:string)  [unwired: 3 in]
                n315 = Number To Fractional String(number=w921) -> (F-format string=w920:string)  [unwired: 3 in]
              }
              n316 = Format Into String(format string="Range: %.3f to %.3f", w889, w888) -> (resulting string=w882:string)  [unwired: 2 in, 1 out]
              n317 = Format Into String(format string="Increment: %.3f", w886) -> (resulting string=w881:string)  [unwired: 2 in, 1 out]
              n318 = Format Into String(format string="Samples: %d", w885) -> (resulting string=w880:string)  [unwired: 2 in, 1 out]
              n319 = Build Array(w882, w881, w880) -> (w879:string[])
              n320 = Build Array(w916, w915) -> (w914:string[][])
              n321 = Transpose 2D Array(2D array=w914) -> (transposed array=w907:string[][])
              n322 = call-dynamic "Append List to Report.vi"("report in"=w894, "list elements"=w879, "list type (ordered)"=enum16{"unordered", "ordered"}."unordered", "error in (no error)"=w893) -> ("report out"=w892:refnum<class "NI_report.lvclass">, "error out"=w891:errorcluster)  [unwired: 8 in, 2 out]
              n323 = call-poly <vilib>:"Append Table to Report.vi"("report in"=w892, "column headers"=string[] ["MICS Power", "Percent Success"], "text data"=w907, "error in (no error)"=w891) -> ("report out"=w906:refnum<class "NI_report.lvclass">, "error out"=w904:errorcluster)  [unwired: 8 in, 2 out]
              n324 = control-ref of="MICS Power Graph"() -> (w913:refnum<vi>)
              n325 = call-dynamic "New Report Line.vi"("report in"=w906, "error in (no error)"=w904) -> ("report out"=w905:refnum<class "NI_report.lvclass">, "error out"=w903:errorcluster)  [unwired: 12 in]
              n326 = To More Generic Class(target class=refnum<vi> refnum ("ctrl reference"), reference=w913) -> (generic class reference=w911:refnum<vi>)
              n327 = call-dynamic "Append Control Image to Report.vi"("report in"=w905, "ctrl reference"=w911, "description"="MICS Power Graph", "error in (no error)"=w903) -> ("report out"=w909:refnum<class "NI_report.lvclass">, "error out"=w908:errorcluster)  [unwired: 8 in, 2 out]
            }
            frame "Generate RF Mapping Section 1" {
              n328 = call-dynamic "Append Horizontal Line to Report.vi"("report in"=w946, "error in (no error)"=w947) -> ("report out"=w944:refnum<class "NI_report.lvclass">, "error out"=w943:errorcluster)  [unwired: 12 in]
              n329 = Unbundle By Name(w940) -> ("Mapping Config.X Range"=w934:cluster{"Min":dbl, "Max":dbl, "Increment":dbl}, "Mapping Config.Y Range"=w933:cluster{"Min":dbl, "Max":dbl, "Increment":dbl}, "Mapping Config.Z Range"=w932:cluster{"Min":dbl, "Max":dbl, "Increment":dbl}, "Mapping Config.Samples"=w929:i32)
              n330 = call "Report - Add Section Header.vi"("report in"=w944, "Heading Size"=enum16{"h1", "h2", "h3"}."h2", "Heading Text"="RF Mapping Results" ("text"), "error in (no error)"=w943) -> ("report out"=w927:refnum<class "NI_report.lvclass">, "error out"=w928:errorcluster)  [unwired: 10 in]
              n331 = Build Array(w934, w933, w932) -> (w931:cluster{"Min":dbl, "Max":dbl, "Increment":dbl}[])
              n332 = for {
                tunnel: [w953] -> w937 mode=indexing
                tunnel: w931 -> [w952] mode=indexing
                tunnel: string[] ["X: ", "Y: ", "Z: "] -> [w948] mode=indexing
                n333 = Unbundle(w952) -> ("Min"=w951:dbl, "Max"=w950:dbl, "Increment"=w949:dbl)
                n334 = Format Into String(format string="%.3f to %.3f, Increment: %.3f", initial string=w948, w951, w950, w949) -> (resulting string=w953:string)  [unwired: 1 in, 1 out]
              }
              n335 = Format Into String(format string="Samples: %d", w929) -> (resulting string=w936:string)  [unwired: 2 in, 1 out]
              n336 = Build Array (concatenate)(w937, w936) -> (w935:string[])
              n337 = call-dynamic "Append List to Report.vi"("report in"=w927, "list elements"=w935, "list type (ordered)"=enum16{"unordered", "ordered"}."unordered", "error in (no error)"=w928) -> ("report out"=w925:refnum<class "NI_report.lvclass">, "error out"=w926:errorcluster)  [unwired: 8 in, 2 out]
            }
            frame "Generate RF Mapping Section 2" {
              n338 = Unbundle By Name(w966) -> ("Mapping Config.X Range"=w961:cluster{"Min":dbl, "Max":dbl, "Increment":dbl}, "Mapping Config.Y Range"=w962:cluster{"Min":dbl, "Max":dbl, "Increment":dbl}, "Mapping Results"=w963:dbl[][][], "Mapping Config.Z Range"=w965:cluster{"Min":dbl, "Max":dbl, "Increment":dbl})
              n339 = call "Range With Increment.vi"("Range"=w961) -> ("Output Array"=w960:dbl[])
              n340 = call "Range With Increment.vi"("Range"=w962) -> ("Output Array"=w959:dbl[])
              n341 = call "Range With Increment.vi"("Range"=w965) -> ("Output Array"=w964:dbl[])
              n342 = for {
                tunnel: w955 -> [w991]
                tunnel: w964 -> [w989] mode=indexing
                tunnel: w963 -> [w987]
                tunnel: w960 -> [w985]
                tunnel: w959 -> [w984]
                tunnel: [w969] -> w958
                shift-right: [w968] -> w957
                shift-left: w956 -> [w992]
                i -> [w986]
                w983 = i16 3 ("precision (6)")
                n343 = Format Into String(format string="z=%.3f", w989) -> (resulting string=w988:string)  [unwired: 2 in, 1 out]
                n344 = Index Array(array=w987, index (dim 2)=w986) -> (element=w977:dbl[][])  [unwired: 2 in]
                n345 = call "Report - Add Section Header.vi"("report in"=w992, "Heading Size"=enum16{"h1", "h2", "h3"}."h3", "Heading Text"=w988, "error in (no error)"=w991) -> ("report out"=w980:refnum<class "NI_report.lvclass">, "error out"=w979:errorcluster)  [unwired: 10 in]
                n346 = Number To Fractional String(number=w985, precision (6)=w983) -> (F-format string=w981:string[])  [unwired: 2 in]
                n347 = Number To Fractional String(number=w984, precision (6)=w983) -> (F-format string=w982:string[])  [unwired: 2 in]
                n348 = call-poly <vilib>:"Append Table to Report.vi"("report in"=w980, "column headers"=w981, "row headers"=w982, "numerical data"=w977, "error in (no error)"=w979) -> ("report out"=w970:refnum<class "NI_report.lvclass">, "error out"=w978:errorcluster)  [unwired: 7 in, 2 out]
                n349 = property on="RF Mapping Graph" class="IntGraph (strict)"(error in=w978, "Val(Sgnl)"=w977) -> (error out=w971:errorcluster)  [unwired: 1 in, 1 out]
                n350 = control-ref of="RF Mapping Graph"() -> (w976:refnum<vi>)
                n351 = call-dynamic "New Report Line.vi"("report in"=w970, "error in (no error)"=w971) -> ("report out"=w973:refnum<class "NI_report.lvclass">, "error out"=w972:errorcluster)  [unwired: 12 in]
                n352 = To More Generic Class(target class=refnum<vi> refnum ("ctrl reference"), reference=w976) -> (generic class reference=w974:refnum<vi>)
                n353 = call-dynamic "Append Control Image to Report.vi"("report in"=w973, "ctrl reference"=w974, "error in (no error)"=w972) -> ("report out"=w968:refnum<class "NI_report.lvclass">, "error out"=w969:errorcluster)  [unwired: 9 in, 2 out]
              }
            }
            frame "Show Report in UI" {
              # "Display the report in app browser"
              n354 = call <vilib>:"Generate Temporary File Path.vi"("error in (no error)"=w1000, "Temporary File Extension (tmp)"="html") -> ("error out"=w1002:errorcluster, "Unique Temporary File Path"=w1003:path)  [unwired: 8 in]
              n355 = Path To String(path=w1003) -> (string=w1004:string)
              n356 = call-dynamic "Save Report to File.vi"("report in"=w999, "report file path"=w1003, "error in (no error)"=w1002) -> ("report out"=w997:refnum<class "NI_report.lvclass">, "error out"=w1001:errorcluster)  [unwired: 11 in]
              n357 = invoke class="IWebBrowser2" method="Navigate"(reference="WebBrowser", error in=w1001, "URL"=w1004) -> (error out=w998:errorcluster)  [unwired: 5 in, 7 out]
            }
          }
        }
        n358 = Bundle By Name(cluster=w774, "Report"=w773) -> (w778:T4)
      }
      frame "Save Report" {
        # "For doge only knows what reason,\nthe prompt VI throws an error when\nthe user cancels"
        n359 = Unbundle By Name(w1020) -> ("Report"=w1011:refnum<class "NI_report.lvclass">, "Previous Start Path"=w1019:path)
        n360 = call "File Dialog"("start path"=w1019, "button label"="Save", "default name"="RF Characterization Report.html", "error in"=w1018, "pattern (all files)"="*.html", "pattern label"="HTML Files") -> ("selected path"=w1012:path, "cancelled"=w1013:bool, "error out"=w1008:errorcluster)  [unwired: 6 in, 1 out]
        n361 = call <vilib>:"Clear Errors.vi"("error in (no error)"=w1008) -> ("error out"=w1007:errorcluster)  [unwired: 6 in]
        n362 = case shown="False" w1013 {
          tunnel: w1007 -> [w1026 w1029]
          tunnel: w1012 -> [w1024 _]
          tunnel: w1011 -> [w1023 _]
          tunnel: [w1022 w1029] -> w1010
          frame False {
            n363 = call-dynamic "Save Report to File.vi"("report in"=w1023, "report file path"=w1024, "prompt to replace? (F)"=TRUE, "error in (no error)"=w1026) -> ("error out"=w1021:errorcluster)  [unwired: 10 in, 1 out]
            n364 = flat-sequence {
              tunnel: [w1027] -> w1022
              tunnel: w1021 -> [w1027]
              frame #0 {
                n365 = One Button Dialog(message="Report saved") -> ()  [unwired: 1 in, 1 out]
              }
            }
          }
          frame True {
          }
        }
      }
      frame "Error" {
        n366 = Variant To Data(error in=w1039, Variant=w1041, type=errorcluster {"status"=FALSE, "code"=0, "source"=""} ("error out")) -> (error out=w1038:errorcluster, data=w1035:errorcluster)
        n367 = Unbundle By Name(w1035) -> ("code"=w1034:i32, "source"=w1033:string)
        n368 = Format Into String(format string="Encountered error (%d) %s\n\nContinue or terminate?", w1034, w1033) -> (resulting string=w1031:string)  [unwired: 2 in, 1 out]
        n369 = Two Button Dialog(message=w1031, 1:"Terminate" ("F button name (\"Cancel\")"), 2:"Continue" ("T button name (\"OK\")")) -> (T button?=w1030:bool)
        n370 = case shown="True" w1030 {
          tunnel: [w1046 w1052] -> w1044
          tunnel: w1043 -> [w1047 w1051]
          tunnel: [w1047 w1050] -> w1042
          tunnel: w1038 -> [w1046 w1048]
          frame True {
          }
          frame False {
            n371 = Enqueue Element(queue=w1051, element=cluster{"State":T2, "Data":variant} {"State"=enum."Shutdown", "Data"=variant}, error in (no error)=w1048) -> (queue out=w1050:refnum<queue>, error out=w1052:errorcluster)  [unwired: 1 in, 1 out]
          }
        }
      }
      frame "Shutdown" {
      }
    }
    n372 = case shown="No Error" w156 {
      selector: w156 -> [w167 w173]
      tunnel: w155 -> [w168 w175]
      tunnel: [w167 w170] -> w154
      tunnel: [w168 w169] -> w153
      frame No Error {
      }
      frame Error {
        n373 = To Variant(anything=w173) -> (Variant=w172:variant)
        n374 = Bundle By Name(cluster=cluster{"State":T2, "Data":variant} {"State"=enum."Error", "Data"=variant} ("element"), "Data"=w172) -> (w171:cluster{"State":T2, "Data":variant})
        n375 = Enqueue Element(queue=w175, element=w171) -> (queue out=w169:refnum<queue>, error out=w170:errorcluster)  [unwired: 2 in, 1 out]
      }
    }
  }
  n376 = Generate User Event(user event=w8, event data cluster=TRUE ("event data"), error in=w9) -> (user event out=w7:refnum<user-event>, error out=w6:errorcluster)
  n377 = Destroy User Event(user event=w7, error in=w6) -> ()  [unwired: 1 out]
